vi "EnFlo_Hub.vi"() -> ()   [LabVIEW 2015]
uses:
  Anemometry Sub Vis/Controls/Launch_controls/Open_Calib.ctl
  Anemometry Sub Vis/Controls/Launch_controls/Open_Meas.ctl
  Anemometry Sub Vis/Controls/Launch_controls/Open_Enter_Temp.ctl
  Anemometry Sub Vis/Controls/Launch_controls/Multi_Run_Prog.ctl
  Anemometry Sub Vis/Controls/Launch_controls/EnFlo_arm.ctl
  Anemometry Sub Vis/Controls/Launch_controls/Fast_FID_Valve.ctl
  Anemometry Sub Vis/Controls/Launch_controls/Disp_Setup.ctl
  Anemometry Sub Vis/Controls/Launch_controls/EnFlo_Tun_Setup.ctl
  Anemometry Sub Vis/Controls/Launch_controls/User_Metadata.ctl
  Anemometry Sub Vis/Controls/Launch_controls/Trav_3D_move.ctl
  Anemometry Sub Vis/Controls/Launch_controls/Trav_Space.ctl
  Anemometry Sub Vis/Controls/Launch_controls/Tunnel_speed.ctl
  Anemometry Sub Vis/Controls/Launch_controls/Client_source_control.ctl
  Anemometry Sub Vis/Controls/Launch_controls/Hydrosonic_Manual.ctl
  Anemometry Sub Vis/Controls/Launch_controls/Preference_Panel.ctl
  Anemometry Sub Vis/Controls/Launch_controls/Hot_wire_Calculator.ctl
  Anemometry Sub Vis/Controls/Launch_controls/RW_X_Parker_Config.ctl
  Anemometry Sub Vis/Controls/Launch_controls/LDA_Alignment.ctl
  Anemometry Sub Vis/Controls/Launch_controls/Named_Serial_Comms.ctl
  Anemometry Sub Vis/Controls/Launch_controls/BSA_data_rates.ctl
  Anemometry Sub Vis/Controls/Launch_controls/Serial_Setup.ctl
  Anemometry Sub Vis/Controls/Launch_controls/Post_Process_icon.ctl
  Anemometry Sub Vis/Controls/Launch_controls/Edit_Ascii_file.ctl
  Anemometry Sub Vis/Controls/Launch_controls/Edit_Raw_DF.ctl
  Anemometry Sub Vis/Controls/Launch_controls/Results_file_plotter.ctl
  Anemometry Sub Vis/Controls/Launch_controls/Serial_Port_Names.ctl
  Anemometry Sub Vis/Controls/Launch_controls/Paul.ctl
  Anemometry Sub Vis/Controls/Launch_controls/Tom.ctl
  Anemometry Sub Vis/Controls/Launch_controls/Scani_Valve.ctl
  Anemometry Sub Vis/Controls/Launch_controls/Edit_sever_Channel.ctl
  Anemometry Sub Vis/Controls/Launch_controls/Day_file_plotter.ctl
  Anemometry Sub Vis/Controls/Launch_controls/Plot_Sever_Data.ctl
  Anemometry Sub Vis/Controls/Launch_controls/Adam_Table.ctl
  Anemometry Sub Vis/Controls/Launch_controls/Active_Channel_Control.ctl
  Anemometry Sub Vis/Controls/Launch_controls/Laser on,off.ctl
  Anemometry Sub Vis/Controls/Launch_controls/Laser set power.ctl
  Anemometry Sub Vis/Controls/Preference_Mode.ctl
  Anemometry Sub Vis/Controls/Post_Process.ctl
  Anemometry Sub Vis/Controls/Server_Comms.ctl
  ADAM Client/Sub VIs/ADAM Controls/Update_scan_value.ctl
  Anemometry Sub Vis/Controls/Setup.ctl
  Anemometry Sub Vis/Gen Trav/Trav_mode.ctl
  Anemometry Sub Vis/Controls/User_Specific_mode.ctl
  Anemometry Sub Vis/File/Setup_Filetype.ctl
  Anemometry Sub Vis/Calibration/Calib_mode.ctl
  Anemometry Sub Vis/Controls/App_Global.ctl
  Anemometry Sub Vis/Globals/Dynamic_call_global.ph.vi
  Anemometry Sub Vis/Globals/Trav_pos_global.vi
  Anemometry Sub Vis/Globals/Constants_global.vi
  Anemometry Sub Vis/Globals/Preference_global.vi
  Anemometry Sub Vis/Acquisition/PWA/PWAtasksGLOBAL.vi
  Anemometry Sub Vis/Globals/Meas_global.vi
  <vilib>/Platform/browser.llb/Open URL in Default Browser (path).vi
  <vilib>/Platform/browser.llb/Open URL in Default Browser (string).vi
  Anemometry Sub Vis/Utilities/Email_transfer_global.vi
  Camera Server/Globals/CamServer global.vi
panel:
  out "CamServer machine name or IP":string="EnFlo-CamServer"
  out "List of ADAM channels to view":string[](array[string])
  out "List of ADAM control channels":string[](array[string])
  out "Analogue Dev Name":string="Dev2"
  out "Numeric":i32
  out "Rig Name":string="EnFlo Tunnel"
  out "All Users":path=path "/System Folder/Preferences/LabVIEW (EnFlo specific)/Meas Setups"
  out "Dummy Measurement":bool
  in  "stop":bool
  in  "Tab Control":T1(tab)
  in  "Tunnel Speed Control":T2
  in  "Traverse Space":T3
  in  "Trav 3D Move":T4 caption="3D Traverse Move"
  in  "User Metadata":T5
  in  "Multi Run Prog":T6
  in  "Enter Temp_Press":T7
  in  "Measurement Prog":T8 caption="Measurement"
  in  "Calibration Prog":T9 caption="Calibration"
  in  "Source Live":bool
  in  "Laser set power":T10
  in  "Laser on/off":T11
  in  "Scani Valve":T12
  in  "LDA Alignment":T13
  in  "Hydrosonic Control":T14
  in  "Fast FID Valve":T15
  in  "Source Control":T16
  in  "Gas Release Setup":T17
  in  "EnFlo Tunnel Setup":T18
  in  "Heater Setup":bool caption="Inlet heater File"
  in  "EnFlo Arm":T19
  in  "EnFlo Tun Display":bool
  in  "Beam Check Positions":bool
  in  "Rig_Control":cluster{"Ch Name":string, "Boolean":bool}[](array[cluster])
  in  "ADAM Channels Control":T20 caption="Change Active Channels"
  in  "ADAM Scan Table":T21 caption="Run ADAM Scan Table"
  in  "Edit Server Channel":T22
  in  "Plot Server Channels":T23 caption="Plot Server Data"
  in  "Day Files Plotter":T24 caption="Plot Data From File"
  out "Current Values":cluster{"Ch Name":string, "Numeric":dbl}[](array[cluster])
  in  "Post_Pro_Results_Hierarchy":bool
  in  "Results File Plotter":T25
  in  "Edit Raw Data Files":T26
  in  "Edit ASCII File":T27
  in  "Post Process Raw Data":T28
  in  "Plot_FFID_Calibs.vi":bool
  in  "Top Level Traverse":bool
  in  "Show Manual Sync":bool
  in  "Sync to server now":bool
  in  "Port Names":T29
  in  "Serial Setup":T30
  in  "LDA Data Rate":T31
  in  "Named Serial Comms":T32
  in  "RW Trav Setup":T33
  in  "Hot Wire Calc":T34
  in  "Preference Panel":T35
  in  "Tom Lawton tlawton@cppwind.com":T36 caption="For -other- support"
  in  "Paul Hayden p.hayden@surrey.ac.uk":T37 caption="For software support"
  in  "Online Manual":bool
  out "VI Name":string
  out "Iterations":i32
  # "Or give us a call on Tel: 01483 689545"
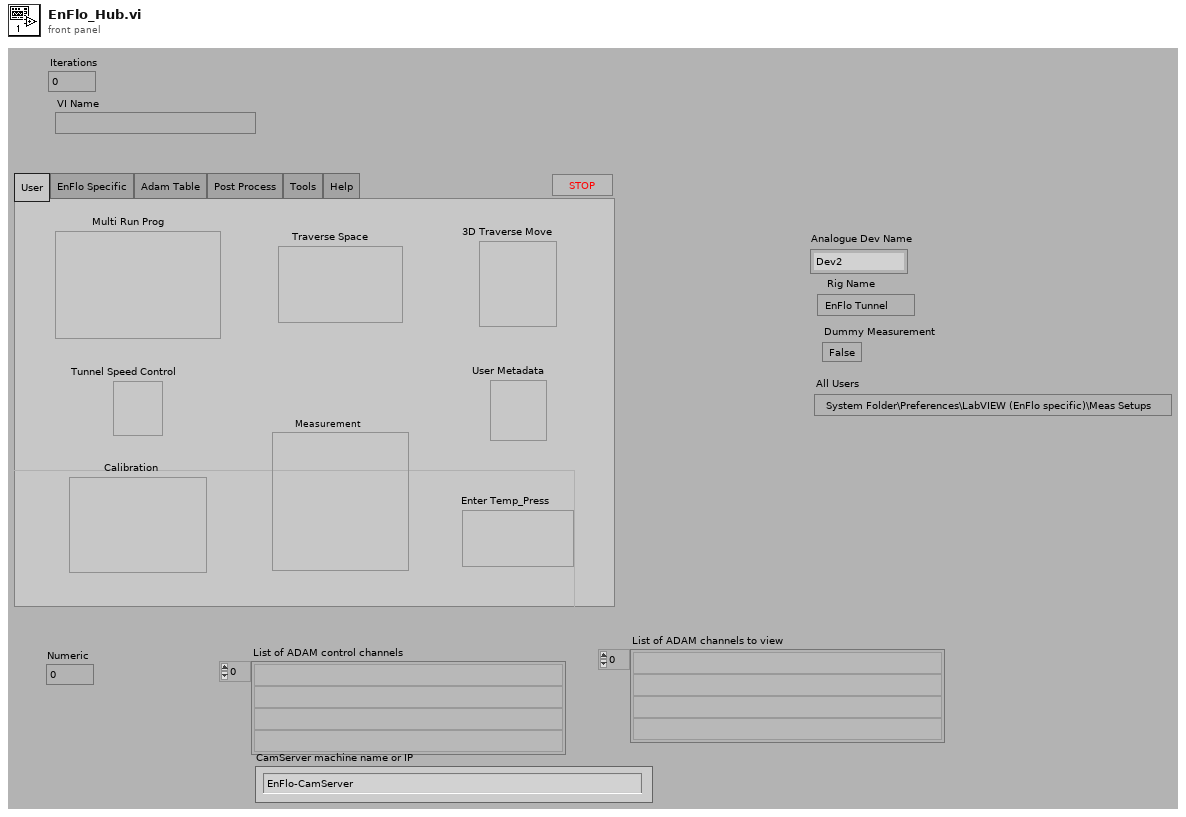
[diagram p1: front panel]
types:
  T1 = enum32{"User", "EnFlo Specific", "Adam Table", "Post Process", "Tools", "Help"}
  T2 = typedef "Tunnel_speed.ctl" = bool
  T3 = typedef "Trav_Space.ctl" = bool
  T4 = typedef "Trav_3D_move.ctl" = bool
  T5 = typedef "User_Metadata.ctl" = bool
  T6 = typedef "Multi_Run_Prog.ctl" = bool
  T7 = typedef "Open_Enter_Temp.ctl" = bool
  T8 = typedef "Open_Meas.ctl" = bool
  T9 = typedef "Open_Calib.ctl" = bool
  T10 = typedef "Laser set power.ctl" = bool
  T11 = typedef "Laser on,off.ctl" = bool
  T12 = typedef "Scani_Valve.ctl" = bool
  T13 = typedef "LDA_Alignment.ctl" = bool
  T14 = typedef "Hydrosonic_Manual.ctl" = bool
  T15 = typedef "Fast_FID_Valve.ctl" = bool
  T16 = typedef "Client_source_control.ctl" = bool
  T17 = typedef "Disp_Setup.ctl" = bool
  T18 = typedef "EnFlo_Tun_Setup.ctl" = bool
  T19 = typedef "EnFlo_arm.ctl" = bool
  T20 = typedef "Active_Channel_Control.ctl" = bool
  T21 = typedef "Adam_Table.ctl" = bool
  T22 = typedef "Edit_sever_Channel.ctl" = bool
  T23 = typedef "Plot_Sever_Data.ctl" = bool
  T24 = typedef "Day_file_plotter.ctl" = bool
  T25 = typedef "Results_file_plotter.ctl" = bool
  T26 = typedef "Edit_Raw_DF.ctl" = bool
  T27 = typedef "Edit_Ascii_file.ctl" = bool
  T28 = typedef "Post_Process_icon.ctl" = bool
  T29 = typedef "Serial_Port_Names.ctl" = bool
  T30 = typedef "Serial_Setup.ctl" = bool
  T31 = typedef "BSA_data_rates.ctl" = bool
  T32 = typedef "Named_Serial_Comms.ctl" = bool
  T33 = typedef "RW_X_Parker_Config.ctl" = bool
  T34 = typedef "Hot_wire_Calculator.ctl" = bool
  T35 = typedef "Preference_Panel.ctl" = bool
  T36 = typedef "Tom.ctl" = bool
  T37 = typedef "Paul.ctl" = bool
  T38 = typedef "Post_Process.ctl" = enum16{"Take New Data", "Post Process Raw Data File"}
  T39 = typedef "Preference_Mode.ctl" = enum16{"Load Preferences from file", "Save Preferences to file", "Load, Edit then Save"}
  T40 = enum32{"User", "EnFlo Lab Specific", "Adam Table", "Post Process", "Tools", "Help"}
  T41 = typedef "Server_Comms.ctl" = enum16{"Server Link Healthy", "Do Not Link To Server"}
  T42 = typedef "Update_scan_value.ctl" = cluster{"Channel Name":string, "New Value":dbl}
  T43 = typedef "Setup.ctl" = enum16{"Run Program", "Show Setup", "Save Current Setup", "Setup Front Panel"}
  T44 = enum16{"Get Channel Names", "Get Current Value", "Update Channel Value", "Update Channel Description"}
  T45 = enum32{"Invalid", "Standard", "Closed", "Hidden", "Minimized", "Maximized"}
  T46 = enum32{"Bad", "Idle", "Run top level", "Running"}
  T47 = enum16{"Load From Excel File", "Save to Excel File"}
  T48 = typedef "User_Specific_mode.ctl" = enum16{"Check VI only", "Run VI"}
  T49 = typedef "Trav_mode.ctl" = enum16{"Move traverse", "Read traverse position", "Teach Position"}
  T50 = typedef "Setup_Filetype.ctl" = enum16{"Measurement Setups", "Calibration Setups", "General", "Results File Plotter Setups", "Speed Calib Tweaks"}
  T51 = enum16{"Load Command File", "Save Command File", "Check Multi Run Prog", "Check Multi Run Prog With Live Moves", "Run Multi Run Prog"}
  T52 = typedef "Calib_mode.ctl" = enum16{"Show Setup", "Take a New Calibration Point", "Refit Curve", "Setup Front Panel"}
  T53 = typedef "App_Global.ctl" = enum16{"Read Global", "Write to Global", "Initialise Array"}
  T54 = typedef "Tunnel_Coordinates.ctl" = enum16{"Work in Tunnel Coordinates", "Work in Model Coordinates"}
  T55 = typedef "App_Ref_Cluster.ctl" = cluster{"Server IP & Port No":string, "Application reference":refnum<vi>}
  T56 = typedef "Ch_description_ADAM.ctl" = cluster{"Ch Name":string, "Type":T57, "Function":T58, "Ch State":T59, "Calibration type":T60, "A":dbl, "B":dbl, "C":dbl, "D":dbl, "Comments":string, "Address":T61, "String":string, "Duty":u16}
  T57 = typedef "Module_type_ADAM.ctl" = string
  T58 = typedef "Function_ADAM.ctl" = enum16{"Analogue Input", "Digital Input", "Event counter", "Event rate", "Analogue Output", "Digital Output", "Relay Output"}
  T59 = typedef "Channel_State.ctl" = enum16{"On", "Off", "Always On", "Always Off"}
  T60 = typedef "Calib_type_ADAM.ctl" = enum16{"Raw", "Bx + A", "Cx^2 + Bx + A", "Dx^3 + Cx^2 + Bx + A", "In Band", "Hi-Tec Q", "Hi-Tec M_dot", "Text"}
  T61 = typedef "Address.ctl" = cluster{"Main":i32, "Ch.":i32, "Sub":i32, "Port Name":string}
  T62 = typedef "Monitor values.ctl" = cluster{"Power (mW)":sgl, "LDD current (A)":sgl, "TEC drive (V)":sgl, "TEC temp. (degC)":sgl, "SHG heater (degC)":sgl, "BRF heater (degC)":sgl}
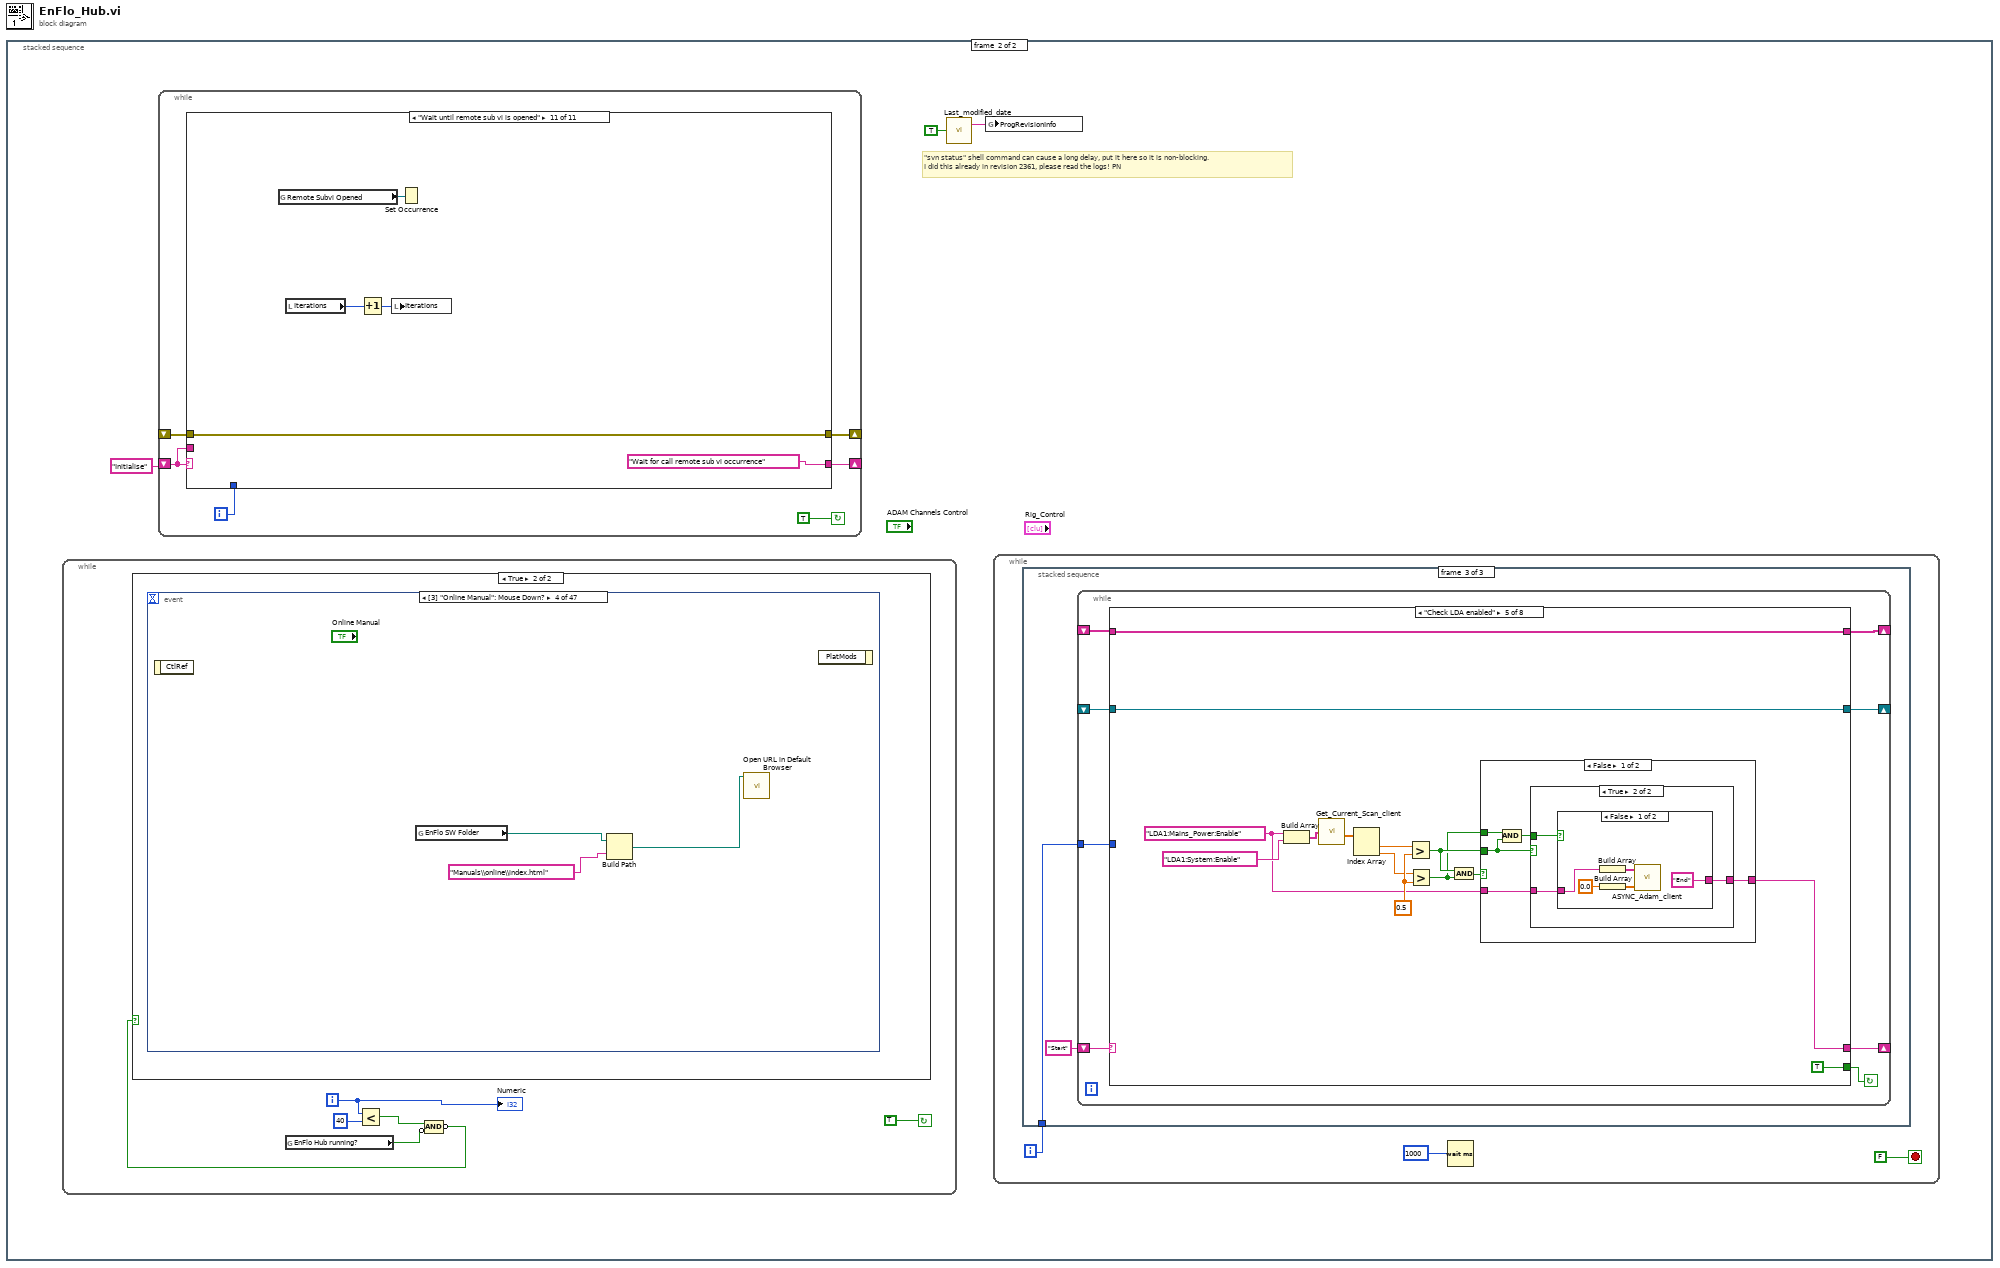
[diagram p0: block diagram]
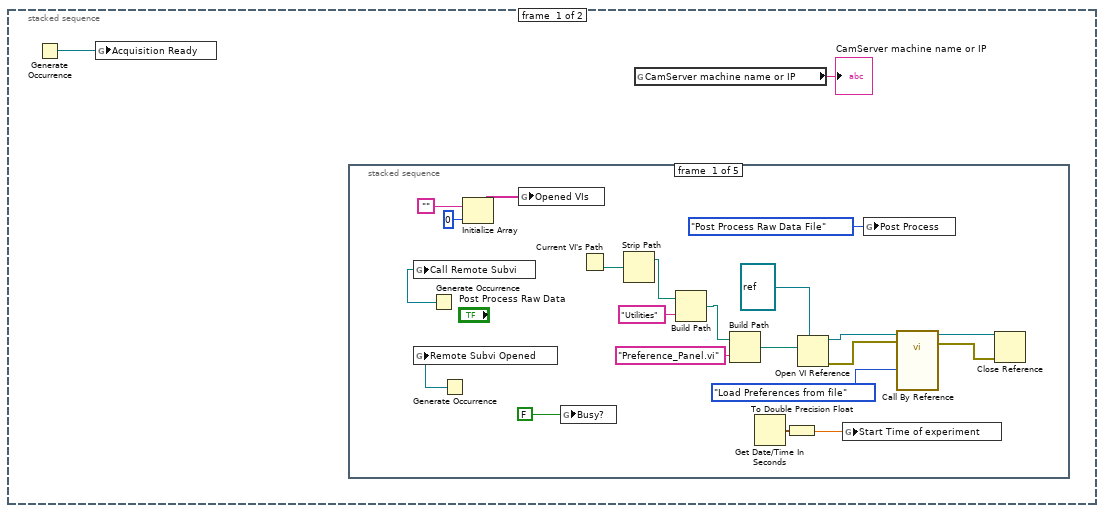
[diagram p2: hidden frame]
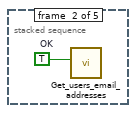
[diagram p3: hidden frame]
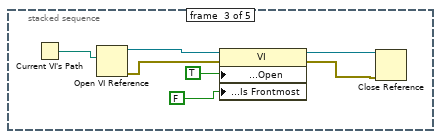
[diagram p4: hidden frame]
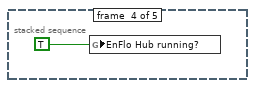
[diagram p5: hidden frame]
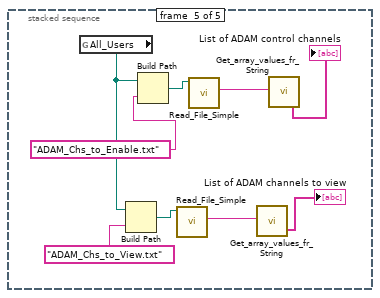
[diagram p6: hidden frame]
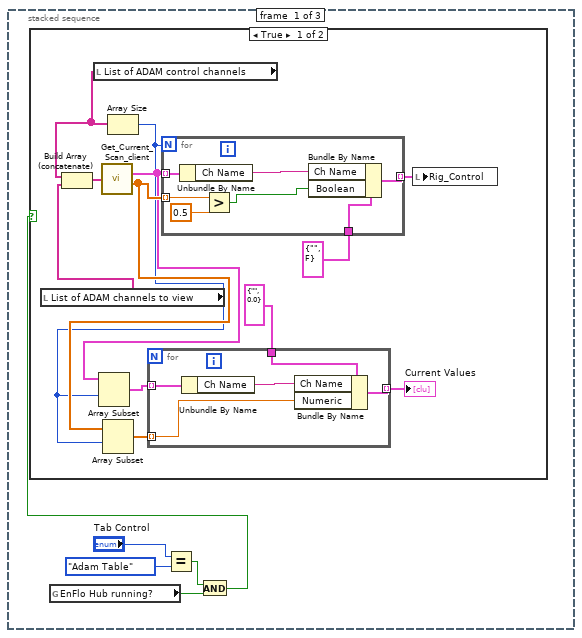
[diagram p7: hidden frame]
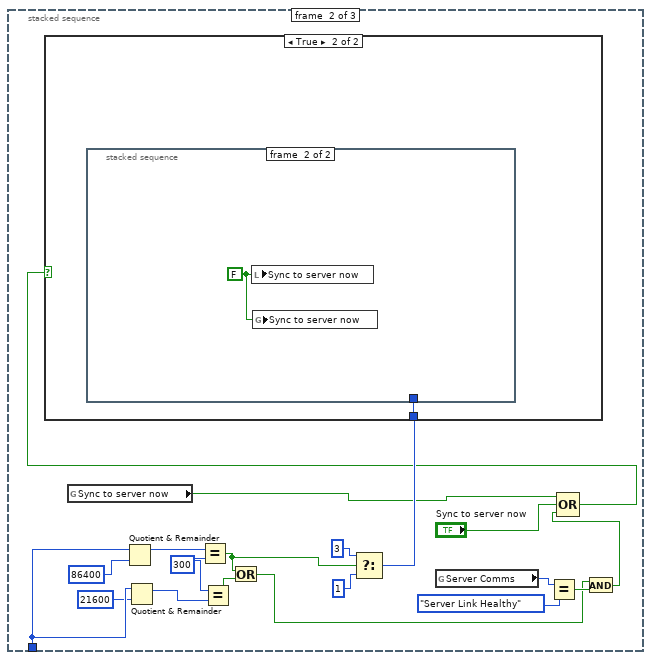
[diagram p9: hidden frame]
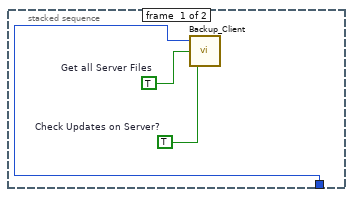
[diagram p11: hidden frame]
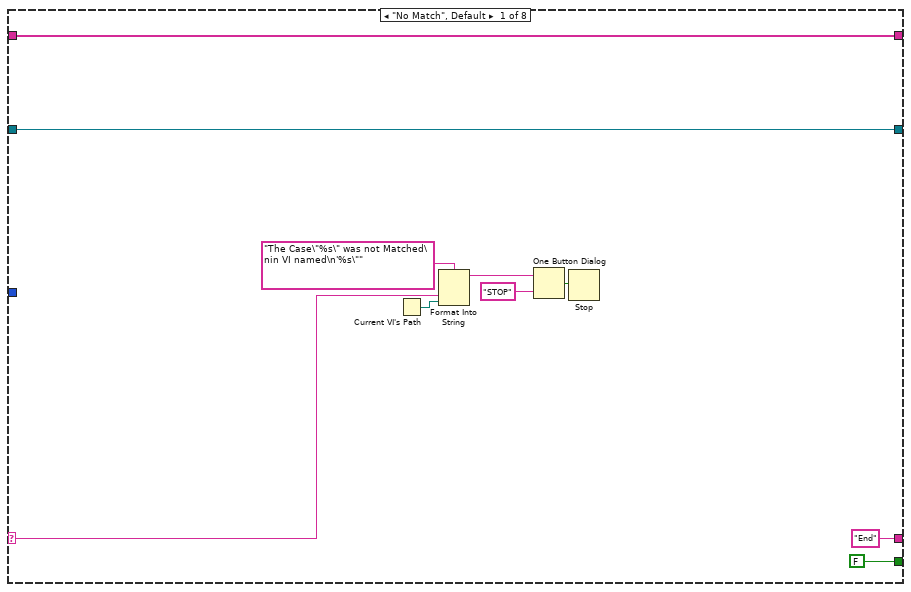
[diagram p12: hidden frame]
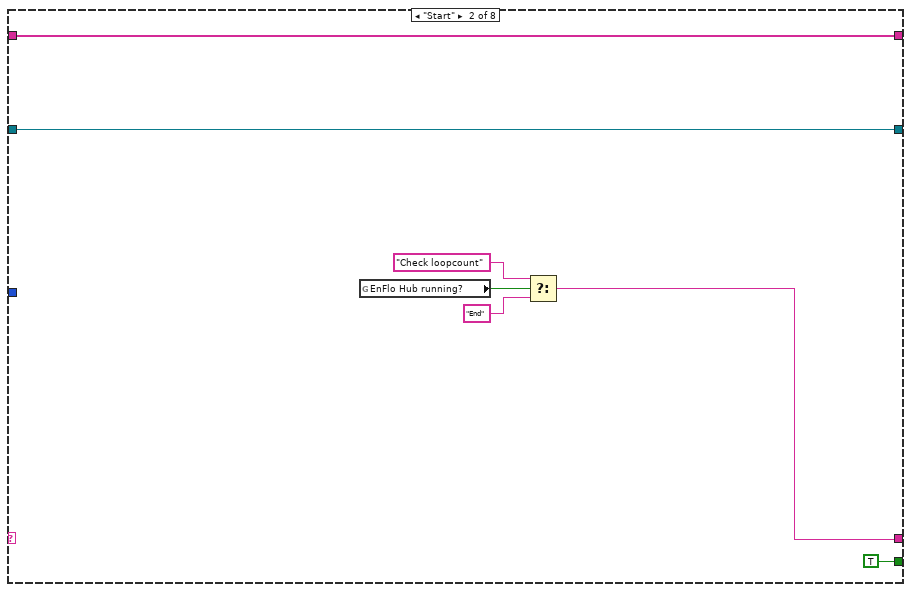
[diagram p13: hidden frame]
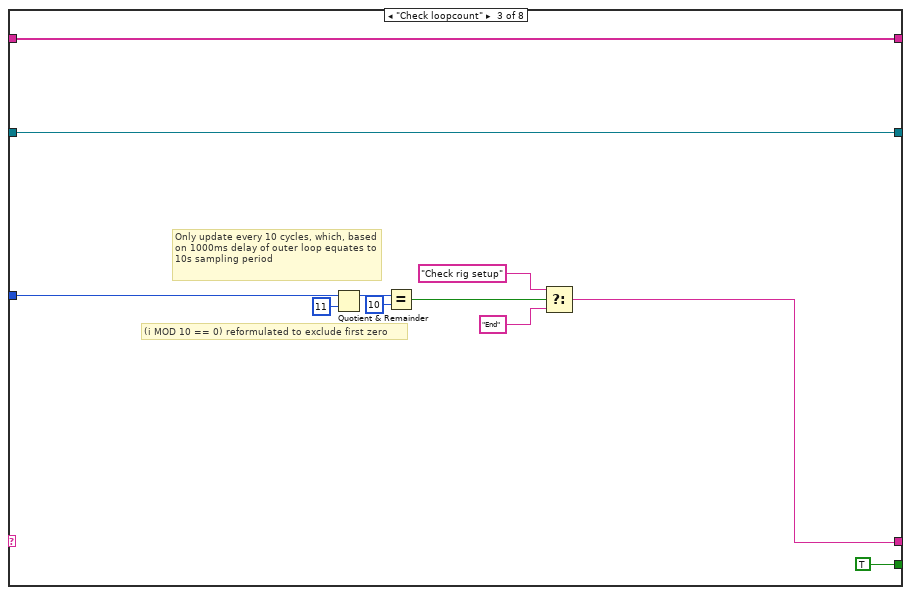
[diagram p14: hidden frame]
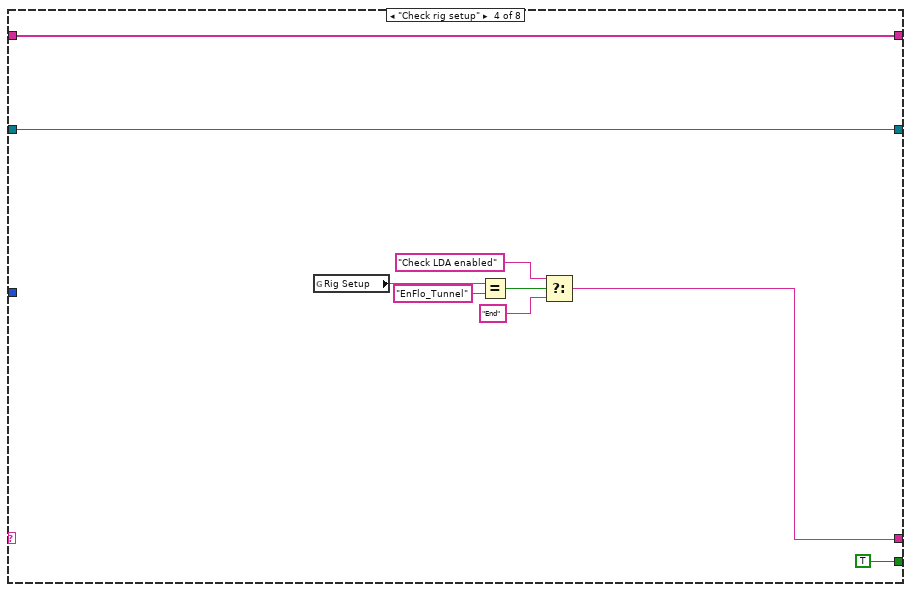
[diagram p15: hidden frame]
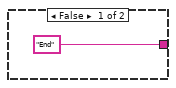
[diagram p16: hidden frame]
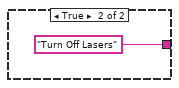
[diagram p17: hidden frame]
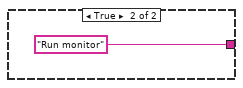
[diagram p18: hidden frame]
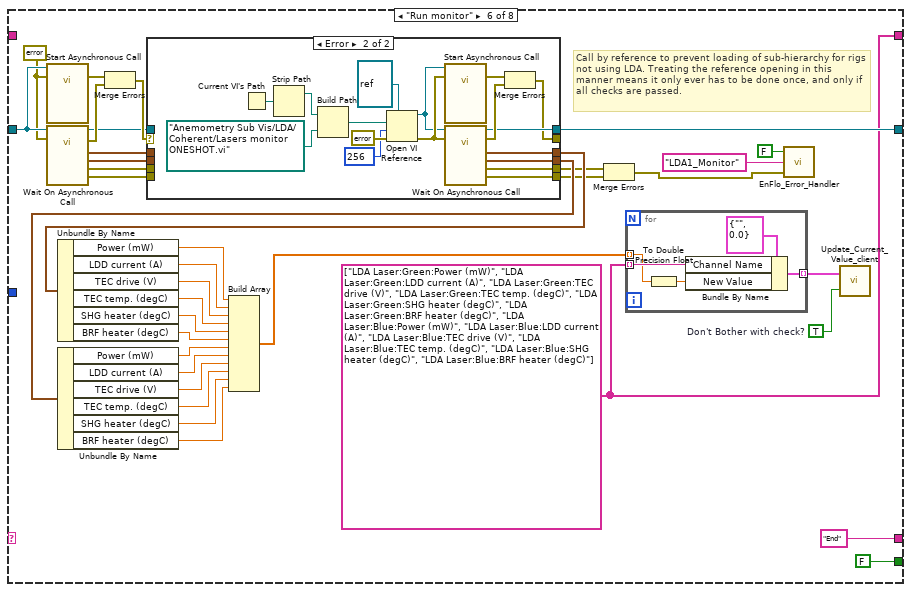
[diagram p19: hidden frame]
diagram:
  n1 = stacked-sequence {
    frame #0 {
      n2 = Generate Occurrence() -> (w2:refnum<k4>)
      n3 = global write "Meas_global.vi" "Acquisition Ready"(w2) -> ()
      n4 = stacked-sequence {
        frame #0 {
          n5 = Generate Occurrence() -> (w23:refnum<k4>)
          n6 = global write "Dynamic_call_global.ph.vi" "Call Remote Subvi"(w23) -> ()
          n7 = Generate Occurrence() -> (w22:refnum<k4>)
          n8 = global write "Dynamic_call_global.ph.vi" "Remote Subvi Opened"(w22) -> ()
          n9 = Initialize Array("", 0) -> (w20:string[])
          n10 = global write "Dynamic_call_global.ph.vi" "Opened VIs"(w20) -> ()
          n11 = global write "Email_transfer_global.vi" "Busy?"(FALSE ("Busy?")) -> ()
          n12 = Current VI's Path() -> (path=w12:path)
          n13 = Strip Path(path=w12) -> (stripped path=w10:path)  [unwired: 1 out]
          n14 = Build Path(base path=w10, name or relative path="Utilities") -> (appended path=w8:path)
          n15 = Build Path(base path=w8, name or relative path="Preference_Panel.vi") -> (appended path=w7:path)
          n16 = Get Date/Time In Seconds() -> (seconds since 1Jan1904=w18:timestamp)
          n17 = To Double Precision Float(number=w18) -> (double precision float=w17:dbl)
          n18 = Open VI Reference(type specifier VI Refnum (for type only)=refnum<vi> refnum, vi path=w7) -> (vi reference=w13:refnum<vi>, error out=w14:errorcluster)  [unwired: 1 in, 3 out]
          n19 = global write "Meas_global.vi" "Start Time of experiment"(w17) -> ()
          n20 = global write "Meas_global.vi" "Post Process"(Post_Process."Post Process Raw Data File" ("Post Process")) -> ()
          n21 = call-by-ref "?"(reference=w13, error in=w14, "Mode"=Preference_Mode."Load Preferences from file") -> (reference out=w15:refnum<vi>, error out=w16:errorcluster)
          n22 = Close Reference(reference=w15, error in (no error)=w16) -> ()  [unwired: 1 out]
        }
        frame #1 {
          w24 = TRUE  # OK
          n23 = call "Get_users_email_addresses.vi"("OK"=w24) -> ()  [unwired: 5 out]
        }
        frame #2 {
          n24 = Current VI's Path() -> (path=w31:path)
          n25 = Open VI Reference(vi path=w31) -> (vi reference=w30:refnum<vi>, error out=w29:errorcluster)  [unwired: 1 in, 4 out]
          n26 = property class="VI"(reference=w30, error in=w29, "Front Panel Window:Open"=TRUE, "Front Panel Window:Is Frontmost"=FALSE) -> (reference out=w28:refnum<vi>, error out=w27:errorcluster)
          n27 = Close Reference(reference=w28, error in (no error)=w27) -> ()  [unwired: 1 out]
        }
        frame #3 {
          n28 = global write "Dynamic_call_global.ph.vi" "EnFlo Hub running?"(TRUE ("EnFlo Hub running?")) -> ()
        }
        frame #4 {
          n29 = global read "Constants_global.vi" "All_Users"() -> (w36:path)
          n30 = Build Path(base path=w36, name or relative path="ADAM_Chs_to_View.txt") -> (appended path=w38:path)
          n31 = Build Path(base path=w36, name or relative path="ADAM_Chs_to_Enable.txt") -> (appended path=w40:path)
          n32 = call "Read_File_Simple.vi"("Filename"=w38) -> ("string"=w37:string)  [unwired: 2 in, 7 out]
          n33 = call "Read_File_Simple.vi"("Filename"=w40) -> ("string"=w41:string)  [unwired: 2 in, 7 out]
          n34 = call "Get_array_values_fr_String.vi"("String Value"=w37) -> ("String array"=→"List of ADAM channels to view":string[])  [unwired: 1 out]
          n35 = call "Get_array_values_fr_String.vi"("String Value"=w41) -> ("String array"=→"List of ADAM control channels":string[])  [unwired: 1 out]
        }
      }
      n36 = global read "CamServer global.vi" "CamServer machine name or IP"() -> (→"CamServer machine name or IP":string)
    }
    frame #1 {
      # "\"svn status\" shell command can cause a long delay, put it here so it is non-blocking.\nI did this already in revision 2361, please read the logs! PN"
      n37 = while {
        i -> [w272]
        stop <- TRUE continue-if-true
        n38 = global read "Dynamic_call_global.ph.vi" "EnFlo Hub running?"() -> (w270:bool)
        n39 = Less?(x=w272, y=40) -> (x < y?=w269:bool)
        n40 = Compound Arithmetic op=AND(w269, invert w270) -> (invert w268:bool)
        n41 = case shown="True" w268 {
          frame False {
            n42 = Wait (ms)(milliseconds to wait=u32 200) -> ()  [unwired: 1 out]
          }
          frame True {
            n43 = event shown="[3] \"Online Manual\": Mouse Down?" {
              selector: _ -> [_ _ _ _ _ _ _ _ _ _ _ _ _ _ _ _ _ _ _ _ _ _ _ _ _ _ _ _ _ _ _ _ _ _ _ _ _ _ _ _ _ _ _ _ _ _ _]
              dyn-events: _ -> [_ _ _ _ _ _ _ _ _ _ _ _ _ _ _ _ _ _ _ _ _ _ _ _ _ _ _ _ _ _ _ _ _ _ _ _ _ _ _ _ _ _ _ _ _ _ _]
              timeout: _ -> [_ _ _ _ _ _ _ _ _ _ _ _ _ _ _ _ _ _ _ _ _ _ _ _ _ _ _ _ _ _ _ _ _ _ _ _ _ _ _ _ _ _ _ _ _ _ _]
              event Mouse Down? {
                w283 = "Measurement.vi" ("name or relative path")
                n44 = event-data() -> ()  [unwired: 2 out]
                n45 = global read "Constants_global.vi" "EnFlo SW Folder"() -> (w286:path)
                n46 = Open VI Reference(vi path=w283) -> (vi reference=w282:refnum<vi>, error out=w281:errorcluster)  [unwired: 1 in, 4 out]
                n47 = Build Path(base path=w286, name or relative path="Anemometry") -> (appended path=w289:path)
                n48 = property class="VI"(reference=w282, error in=w281, "Front Panel Window:Open"=TRUE) -> (reference out=w279:refnum<vi>, error out=w280:errorcluster)
                n49 = Build Path(base path=w289, name or relative path=w283) -> (appended path=w287:path)
                n50 = global read "Preference_global.vi" "Rig Setup"() -> (w277:string)
                n51 = Close Reference(reference=w279, error in (no error)=w280) -> (error out=w278:errorcluster)
                n52 = Unbundle By Name(w278) -> ("status"=w288:bool)
                n53 = Equal?(x="Post_Processing_Machine" ("Rig Setup"), y=w277) -> (x = y?=w275:bool)
                n54 = case shown="True" w288 {
                  tunnel: w287 -> [_ w292]
                  tunnel: w278 -> [_ _]
                  tunnel: w275 -> [_ w291]
                  frame False {
                  }
                  frame True {
                    n55 = stacked-sequence {
                      tunnel: w292 -> [w302 _]
                      tunnel: w291 -> [w293 _]
                      frame #0 {
                        n56 = Open VI Reference(type specifier VI Refnum (for type only)=refnum<vi> refnum, vi path=w302) -> (vi reference=w300:refnum<vi>, error out=w299:errorcluster)  [unwired: 1 in, 3 out]
                        n57 = property class="VI Interface Type 2"(reference=w300, error in=w299, "Front Panel Window:Open"=TRUE) -> (reference out=w295:refnum<vi>, error out=w294:errorcluster)
                        n58 = case shown="False" w293 {
                          tunnel: [w308 w310] -> w298
                          tunnel: [w307 w309] -> w297
                          tunnel: w295 -> [w306 w310]
                          tunnel: w294 -> [w305 w309]
                          frame False {
                            n59 = call-by-ref "?"(reference=w306, error in=w305, "setup"=Setup."Setup Front Panel", "Post Process"=Post_Process."Take New Data") -> (reference out=w308:refnum<vi>, error out=w307:errorcluster)  [unwired: 16 in, 2 out]
                          }
                          frame True {
                          }
                        }
                        n60 = Close Reference(reference=w298, error in (no error)=w297) -> ()  [unwired: 1 out]
                      }
                      frame #1 {
                        n61 = global write "Meas_global.vi" "Post Process"(Post_Process."Post Process Raw Data File" ("Post Process")) -> ()
                      }
                    }
                  }
                }
                n62 = event-data("Discard?"=TRUE) -> ()  [unwired: 1 in, 2 out]
              }
              event Mouse Down? {
                n63 = event-data() -> ()  [unwired: 2 out]
                n64 = call-poly <vilib>:"Open URL in Default Browser.vi"("URL"="Mailto:tlawton@cppwind.com") -> ()  [unwired: 1 in, 6 out]
                n65 = event-data() -> ()  [unwired: 1 in, 5 out]
              }
              event Mouse Down? {
                n66 = event-data() -> ()  [unwired: 5 out]
                n67 = call-poly <vilib>:"Open URL in Default Browser.vi"("URL"="Mailto:p.hayden@surrey.ac.uk") -> ()  [unwired: 1 in, 6 out]
                n68 = event-data() -> ()  [unwired: 1 in, 2 out]
              }
              event "Online Manual": Mouse Down? {
                n69 = event-data() -> ()  [unwired: 2 out]
                n70 = global read "Constants_global.vi" "EnFlo SW Folder"() -> (w316:path)
                n71 = Build Path(base path=w316, name or relative path="Manuals\\online\\index.html" ("URL")) -> (appended path=w314:path)
                n72 = call-poly <vilib>:"Open URL in Default Browser.vi"("path"=w314) -> ()  [unwired: 1 in, 6 out]
                n73 = event-data() -> ()  [unwired: 1 in, 2 out]
              }
              event Mouse Down? {
                n74 = event-data() -> ()  [unwired: 9 out]
                n75 = global read "Constants_global.vi" "EnFlo SW Folder"() -> (w317:path)
                n76 = Build Path(base path=w317, name or relative path=path "ADAM Client/ADAM client VIs/ScaniValve_client.vi") -> (appended path=w320:path)
                n77 = call "Open_Close_Front_Panel.ph.vi"("Front Panel Window:Open"=TRUE, "VI path"=w320) -> ()  [unwired: 2 out]
                n78 = event-data() -> ()  [unwired: 1 in, 5 out]
              }
              event Mouse Down? {
                n79 = event-data() -> ()  [unwired: 9 out]
                n80 = global read "Constants_global.vi" "EnFlo SW Folder"() -> (w321:path)
                n81 = Build Path(base path=w321, name or relative path=path "Anemometry/Anemometry Sub Vis/LDA/Coherent/Laser power on,off (simple).vi") -> (appended path=w324:path)
                n82 = call "Open_Close_Front_Panel.ph.vi"("Front Panel Window:Open"=TRUE, "VI path"=w324) -> ()  [unwired: 2 out]
                n83 = event-data() -> ()  [unwired: 2 in, 1 out]
              }
              event "Source Live": Value Change {
                n84 = event-data() -> ()  [unwired: 7 out]
                n85 = flat-sequence {
                  frame #0 {
                    n86 = global read "Constants_global.vi" "EnFlo SW Folder"() -> (w325:path)
                    n87 = Build Path(base path=w325, name or relative path=path "ADAM Serial/Instrument drivers/Arduino/Source_Live_Control.vi") -> (appended path=w328:path)
                    n88 = call "Open_Close_Front_Panel.ph.vi"("Front Panel Window:Open"=TRUE, "VI path"=w328) -> ()  [unwired: 2 out]
                  }
                  frame #1 {
                    n89 = local write "Source Live"(FALSE) -> ()
                  }
                }
              }
              event Mouse Down? {
                n90 = event-data() -> ()  [unwired: 9 out]
                n91 = global read "Constants_global.vi" "EnFlo SW Folder"() -> (w330:path)
                n92 = Build Path(base path=w330, name or relative path=path "Anemometry/Anemometry Sub Vis/LDA/Coherent/Set lasers power.vi") -> (appended path=w333:path)
                n93 = call "Open_Close_Front_Panel.ph.vi"("Front Panel Window:Open"=TRUE, "VI path"=w333) -> ()  [unwired: 2 out]
                n94 = event-data() -> ()  [unwired: 2 in, 1 out]
              }
              event Mouse Down? {
                n95 = event-data() -> ()  [unwired: 5 out]
                n96 = global read "Constants_global.vi" "EnFlo SW Folder"() -> (w334:path)
                n97 = Build Path(base path=w334, name or relative path=path "ADAM Client/ADAM client VIs/Day_File_Plotter.vi") -> (appended path=w340:path)
                n98 = Open VI Reference(vi path=w340) -> (vi reference=w341:refnum<vi>, error out=w343:errorcluster)  [unwired: 2 in, 3 out]
                n99 = property class="VI"(reference=w341, error in=w343, "Front Panel Window:Open"=TRUE) -> (reference out=w345:refnum<vi>, error out=w344:errorcluster)
                n100 = invoke class="VI" method="Run VI"(reference=w345, error in=w344, "Wait until done"=FALSE, "Auto Dispose Ref"=TRUE) -> (reference out=w336:refnum<vi>, error out=w337:errorcluster)  [unwired: 1 in, 3 out]
                n101 = Close Reference(reference=w336, error in (no error)=w337) -> ()  [unwired: 1 out]
                n102 = event-data() -> ()  [unwired: 1 in, 4 out]
              }
              event Mouse Down? {
                n103 = event-data() -> ()  [unwired: 5 out]
                n104 = global read "Constants_global.vi" "EnFlo SW Folder"() -> (w346:path)
                n105 = Build Path(base path=w346, name or relative path=path "ADAM Serial/Serial Link Layer/Port_Names.vi") -> (appended path=w348:path)
                n106 = Open VI Reference(vi path=w348) -> (vi reference=w353:refnum<vi>, error out=w354:errorcluster)  [unwired: 1 in, 4 out]
                n107 = invoke class="VI" method="Run VI"(reference=w353, error in=w354, "Wait until done"=TRUE, "Auto Dispose Ref"=TRUE) -> (reference out=w349:refnum<vi>, error out=w350:errorcluster)  [unwired: 1 in, 3 out]
                n108 = Close Reference(reference=w349, error in (no error)=w350) -> ()  [unwired: 1 out]
                n109 = event-data() -> ()  [unwired: 1 in, 5 out]
              }
              event Mouse Down? {
                n110 = event-data() -> ()  [unwired: 5 out]
                n111 = global read "Constants_global.vi" "EnFlo SW Folder"() -> (w355:path)
                n112 = Build Path(base path=w355, name or relative path=path "Data plotting/Results_file_Plotter.vi") -> (appended path=w358:path)
                n113 = Open VI Reference(vi path=w358) -> (vi reference=w360:refnum<vi>, error out=w357:errorcluster)  [unwired: 1 in, 4 out]
                n114 = property class="VI"(reference=w360, error in=w357, "Front Panel Window:Open"=TRUE) -> (reference out=w361:refnum<vi>, error out=w362:errorcluster)
                n115 = invoke class="VI" method="Run VI"(reference=w361, error in=w362, "Wait until done"=FALSE, "Auto Dispose Ref"=TRUE) -> (reference out=w363:refnum<vi>, error out=w364:errorcluster)  [unwired: 1 in, 3 out]
                n116 = Close Reference(reference=w363, error in (no error)=w364) -> ()  [unwired: 1 out]
                n117 = event-data() -> ()  [unwired: 1 in, 5 out]
              }
              event Mouse Down? {
                n118 = event-data() -> ()  [unwired: 5 out]
                n119 = global read "Constants_global.vi" "EnFlo SW Folder"() -> (w367:path)
                n120 = Build Path(base path=w367, name or relative path=path "Anemometry/Utilities/Post_Process_Raw_data.vi") -> (appended path=w369:path)
                n121 = call "Open_Close_Front_Panel.ph.vi"("Front Panel Window:Open"=TRUE, "VI path"=w369) -> ()  [unwired: 2 out]
                n122 = event-data() -> ()  [unwired: 1 in, 5 out]
              }
              event Mouse Down? {
                n123 = event-data() -> ()  [unwired: 5 out]
                n124 = global read "Constants_global.vi" "EnFlo SW Folder"() -> (w371:path)
                n125 = Build Path(base path=w371, name or relative path=path "Anemometry/Anemometry Sub Vis/Data_plotting_vis/Edit_Raw_DF_Header.vi") -> (appended path=w373:path)
                n126 = call "Open_Close_Front_Panel.ph.vi"("Front Panel Window:Open"=TRUE, "VI path"=w373) -> ()  [unwired: 2 out]
                n127 = event-data() -> ()  [unwired: 1 in, 5 out]
              }
              event Mouse Down? {
                n128 = event-data() -> ()  [unwired: 5 out]
                n129 = global read "Constants_global.vi" "EnFlo SW Folder"() -> (w375:path)
                n130 = Build Path(base path=w375, name or relative path=path "ADAM Serial/Serial Link Layer/Serial_Setup.vi") -> (appended path=w377:path)
                n131 = Open VI Reference(vi path=w377) -> (vi reference=w382:refnum<vi>, error out=w383:errorcluster)  [unwired: 1 in, 4 out]
                n132 = invoke class="VI" method="Run VI"(reference=w382, error in=w383, "Wait until done"=TRUE, "Auto Dispose Ref"=TRUE) -> (reference out=w378:refnum<vi>, error out=w379:errorcluster)  [unwired: 1 in, 3 out]
                n133 = Close Reference(reference=w378, error in (no error)=w379) -> ()  [unwired: 1 out]
                n134 = event-data() -> ()  [unwired: 1 in, 2 out]
              }
              event Mouse Down? {
                n135 = event-data() -> ()  [unwired: 5 out]
                n136 = global read "Constants_global.vi" "EnFlo SW Folder"() -> (w385:path)
                n137 = Build Path(base path=w385, name or relative path=path "ADAM Serial/Serial Link Layer/Named_Serial_Comms.vi") -> (appended path=w387:path)
                n138 = call "Open_Close_Front_Panel.ph.vi"("Front Panel Window:Open"=TRUE, "VI path"=w387) -> ()  [unwired: 2 out]
                n139 = event-data() -> ()  [unwired: 1 in, 5 out]
              }
              event Mouse Down? {
                n140 = event-data() -> ()  [unwired: 5 out]
                n141 = global read "Constants_global.vi" "EnFlo SW Folder"() -> (w388:path)
                n142 = Build Path(base path=w388, name or relative path=path "Anemometry/Anemometry Sub Vis/LDA/LDA_data_rate.vi") -> (appended path=w390:path)
                n143 = call "Open_Close_Front_Panel.ph.vi"("Front Panel Window:Open"=TRUE, "VI path"=w390) -> ()  [unwired: 2 out]
                n144 = event-data() -> ()  [unwired: 1 in, 2 out]
              }
              event Mouse Down? {
                n145 = event-data() -> ()  [unwired: 5 out]
                n146 = global read "Constants_global.vi" "EnFlo SW Folder"() -> (w402:path)
                n147 = Build Path(base path=w402, name or relative path=path "ADAM Client/ADAM client VIs/Control_Channel_Status.vi") -> (appended path=w392:path)
                n148 = Open VI Reference(vi path=w392) -> (vi reference=w395:refnum<vi>, error out=w393:errorcluster)  [unwired: 1 in, 4 out]
                n149 = property class="VI"(reference=w395, error in=w393, "Front Panel Window:Open"=TRUE) -> (reference out=w396:refnum<vi>, error out=w397:errorcluster)
                n150 = invoke class="VI" method="Run VI"(reference=w396, error in=w397, "Wait until done"=FALSE, "Auto Dispose Ref"=TRUE) -> (reference out=w398:refnum<vi>, error out=w399:errorcluster)  [unwired: 1 in, 3 out]
                n151 = Close Reference(reference=w398, error in (no error)=w399) -> ()  [unwired: 1 out]
                n152 = event-data() -> ()  [unwired: 1 in, 2 out]
              }
              event Mouse Down? {
                n153 = event-data() -> ()  [unwired: 5 out]
                n154 = global read "Constants_global.vi" "EnFlo SW Folder"() -> (w404:path)
                n155 = Build Path(base path=w404, name or relative path=path "Anemometry/Utilities/LDA_Beam_Alignment.vi") -> (appended path=w406:path)
                n156 = call "Open_Close_Front_Panel.ph.vi"("Front Panel Window:Open"=TRUE, "VI path"=w406) -> ()  [unwired: 2 out]
                n157 = event-data() -> ()  [unwired: 1 in, 5 out]
              }
              event Mouse Down? {
                w409 = FALSE  # Wait until done
                n158 = event-data() -> ()  [unwired: 5 out]
                n159 = call "Run_Enter_Temp.vi"("Wait until done"=w409) -> ()  [unwired: 1 out]
                n160 = event-data("Discard?"=TRUE) -> ()  [unwired: 1 in, 4 out]
              }
              event Mouse Down? {
                n161 = event-data() -> ()  [unwired: 5 out]
                n162 = global read "Constants_global.vi" "EnFlo SW Folder"() -> (w410:path)
                n163 = Build Path(base path=w410, name or relative path=path "Anemometry/Utilities/Edit_ASCI_file.vi") -> (appended path=w413:path)
                n164 = call "Open_Close_Front_Panel.ph.vi"("Front Panel Window:Open"=TRUE, "VI path"=w413) -> ()  [unwired: 2 out]
                n165 = event-data() -> ()  [unwired: 1 in, 5 out]
              }
              event "Heater Setup": Mouse Down? {
                n166 = event-data() -> ()  [unwired: 5 out]
                n167 = global read "Constants_global.vi" "EnFlo SW Folder"() -> (w414:path)
                n168 = Build Path(base path=w414, name or relative path=path "Anemometry/Utilities/Create_Heater_Setpoints_File.vi") -> (appended path=w417:path)
                n169 = call "Open_Close_Front_Panel.ph.vi"("Front Panel Window:Open"=TRUE, "VI path"=w417) -> ()  [unwired: 2 out]
                n170 = event-data() -> ()  [unwired: 1 in, 5 out]
              }
              event Mouse Down? {
                n171 = event-data() -> ()  [unwired: 5 out]
                n172 = global read "Constants_global.vi" "EnFlo SW Folder"() -> (w418:path)
                n173 = Build Path(base path=w418, name or relative path=path "ADAM Client/Sub VIs/Gas_Release_Control.vi") -> (appended path=w421:path)
                n174 = call "Open_Close_Front_Panel.ph.vi"("Front Panel Window:Open"=TRUE, "VI path"=w421) -> ()  [unwired: 2 out]
                n175 = event-data() -> ()  [unwired: 1 in, 5 out]
              }
              event Mouse Down? {
                n176 = event-data() -> ()  [unwired: 5 out]
                n177 = global read "Constants_global.vi" "EnFlo SW Folder"() -> (w422:path)
                n178 = Build Path(base path=w422, name or relative path=path "ADAM Client/ADAM client VIs/Edit_Server_Channel.vi") -> (appended path=w432:path)
                n179 = Open VI Reference(type specifier VI Refnum (for type only)=refnum<vi> refnum, vi path=w432) -> (vi reference=w425:refnum<vi>, error out=w426:errorcluster)  [unwired: 1 in, 3 out]
                n180 = property class="VI Interface Type 3"(reference=w425, error in=w426, "Front Panel Window:Open"=TRUE) -> (reference out=w428:refnum<vi>, error out=w429:errorcluster)
                n181 = call-by-ref "?"(reference=w428, error in=w429, "Mode"=T44."Get Channel Names") -> (reference out=w430:refnum<vi>, error out=w431:errorcluster)  [unwired: 5 in]
                n182 = Close Reference(reference=w430, error in (no error)=w431) -> ()  [unwired: 1 out]
                n183 = event-data() -> ()  [unwired: 1 in, 5 out]
              }
              event "EnFlo Tun Display": Mouse Down? {
                n184 = event-data() -> ()  [unwired: 9 out]
                n185 = global read "Constants_global.vi" "EnFlo SW Folder"() -> (w445:path)
                n186 = Build Path(base path=w445, name or relative path=path "Anemometry/Utilities/EnFlo_Tunnel_Display.vi") -> (appended path=w440:path)
                n187 = Open VI Reference(vi path=w440) -> (vi reference=w439:refnum<vi>, error out=w438:errorcluster)  [unwired: 5 in]
                n188 = invoke class="VI" method="FP.Open"(reference=w439, error in=w438, "Activate"=TRUE ("Activate?"), "State"=T45."Standard") -> (reference out=w437:refnum<vi>, error out=w436:errorcluster)  [unwired: 1 in, 3 out]
                n189 = invoke class="VI" method="Run VI"(reference=w437, error in=w436, "Wait until done"=FALSE ("Wait Until Done"), "Auto Dispose Ref"=FALSE ("Wait until done")) -> (reference out=w441:refnum<vi>, error out=w442:errorcluster)  [unwired: 1 in, 3 out]
                n190 = Close Reference(reference=w441, error in (no error)=w442) -> ()  [unwired: 1 out]
                n191 = event-data() -> ()  [unwired: 5 in, 1 out]
              }
              event Mouse Down? {
                n192 = event-data() -> ()  [unwired: 5 out]
                n193 = global read "Constants_global.vi" "EnFlo SW Folder"() -> (w447:path)
                n194 = Build Path(base path=w447, name or relative path=path "ADAM Client/ADAM client VIs/Set_Tunnel_Speed.vi") -> (appended path=w450:path)
                n195 = call "Open_Close_Front_Panel.ph.vi"("Front Panel Window:Open"=TRUE, "VI path"=w450) -> ()  [unwired: 2 out]
                n196 = event-data() -> ()  [unwired: 1 in, 5 out]
              }
              event Mouse Down? {
                n197 = event-data() -> ()  [unwired: 5 out]
                n198 = global read "Constants_global.vi" "EnFlo SW Folder"() -> (w451:path)
                n199 = Build Path(base path=w451, name or relative path=path "ADAM Client/ADAM client VIs/Plot_Server_Data.vi") -> (appended path=w454:path)
                n200 = Open VI Reference(vi path=w454) -> (vi reference=w456:refnum<vi>, error out=w453:errorcluster)  [unwired: 1 in, 4 out]
                n201 = property class="VI"(reference=w456, error in=w453, "Front Panel Window:Open"=TRUE) -> (reference out=w457:refnum<vi>, error out=w458:errorcluster)
                n202 = invoke class="VI" method="Run VI"(reference=w457, error in=w458, "Wait until done"=FALSE, "Auto Dispose Ref"=TRUE) -> (reference out=w459:refnum<vi>, error out=w460:errorcluster)  [unwired: 1 in, 3 out]
                n203 = Close Reference(reference=w459, error in (no error)=w460) -> ()  [unwired: 1 out]
                n204 = event-data() -> ()  [unwired: 1 in, 5 out]
              }
              event Mouse Down? {
                n205 = event-data() -> ()  [unwired: 5 out]
                n206 = global read "Constants_global.vi" "EnFlo SW Folder"() -> (w470:path)
                n207 = Build Path(base path=w470, name or relative path=path "ADAM Server/ADAM_scan_table.vi") -> (appended path=w468:path)
                n208 = Open VI Reference(vi path=w468) -> (vi reference=w471:refnum<vi>, error out=w472:errorcluster)  [unwired: 1 in, 4 out]
                n209 = property class="VI"(reference=w471, error in=w472) -> (reference out=w466:refnum<vi>, error out=w465:errorcluster, "Execution:State"=w473:T46)
                n210 = Equal?(x=w473, y=T46."Run top level" ("Execution:State")) -> (x = y?=w467:bool)
                n211 = case shown="False" w467 {
                  tunnel: w466 -> [w478 w495]
                  tunnel: w465 -> [w477 w494]
                  tunnel: [w476 w495] -> w464
                  tunnel: [w475 w494] -> w463
                  frame False {
                    n212 = Two Button Dialog(message="Are you sure that you want to Run the ADAM Scan table on this machine?", 1:"Run" ("F button name (\"Cancel\")"), 2:"Cancel" ("T button name (\"OK\")")) -> (T button?=w479:bool)
                    n213 = case shown="False" w479 {
                      tunnel: w478 -> [w486 w493]
                      tunnel: w477 -> [w485 w492]
                      tunnel: [w484 w493] -> w476
                      tunnel: [w483 w492] -> w475
                      frame False {
                        n214 = property class="VI"(reference=w486, error in=w485, "Front Panel Window:Open"=TRUE) -> (reference out=w490:refnum<vi>, error out=w489:errorcluster)
                        n215 = invoke class="VI" method="Run VI"(reference=w490, error in=w489, "Wait until done"=FALSE, "Auto Dispose Ref"=TRUE) -> (reference out=w484:refnum<vi>, error out=w483:errorcluster)  [unwired: 1 in, 3 out]
                      }
                      frame True {
                      }
                    }
                  }
                  frame True {
                  }
                }
                n216 = event-data() -> ()  [unwired: 1 in, 2 out]
                n217 = Close Reference(reference=w464, error in (no error)=w463) -> ()  [unwired: 1 out]
              }
              event Mouse Down? {
                n218 = event-data() -> ()  [unwired: 5 out]
                n219 = global read "Constants_global.vi" "EnFlo SW Folder"() -> (w498:path)
                n220 = Build Path(base path=w498, name or relative path=path "ADAM Serial/Instrument drivers/Traverses/~subVIs/Read_Write_Trav_Config.vi") -> (appended path=w499:path)
                n221 = Build Path(base path=w498, name or relative path=path "ADAM Serial/Instrument drivers/Traverses/~subVIs/DriveConfigGlobal.vi") -> (appended path=w500:path)
                n222 = flat-sequence {
                  tunnel: w500 -> [w501]
                  tunnel: w499 -> [w503]
                  frame #0 {
                    n223 = call "Open_Close_Front_Panel.ph.vi"("Front Panel Window:Open"=TRUE, "VI path"=w501) -> ()  [unwired: 2 out]
                  }
                  frame #1 {
                    n224 = call "Open_Close_Front_Panel.ph.vi"("Front Panel Window:Open"=TRUE, "VI path"=w503) -> ()  [unwired: 2 out]
                  }
                }
                n225 = event-data() -> ()  [unwired: 1 in, 5 out]
              }
              event Mouse Down? {
                n226 = event-data() -> ()  [unwired: 5 out]
                n227 = global read "Constants_global.vi" "EnFlo SW Folder"() -> (w505:path)
                n228 = Build Path(base path=w505, name or relative path=path "Anemometry/Utilities/Hot_wire_Calculator.vi") -> (appended path=w508:path)
                n229 = call "Open_Close_Front_Panel.ph.vi"("Front Panel Window:Open"=TRUE, "VI path"=w508) -> ()  [unwired: 2 out]
                n230 = event-data() -> ()  [unwired: 1 in, 5 out]
              }
              event "Show Manual Sync": Mouse Down {
                n231 = event-data() -> ()  [unwired: 9 out]
                n232 = global read "Constants_global.vi" "EnFlo SW Folder"() -> (w509:path)
                n233 = Build Path(base path=w509, name or relative path=path "Anemometry/Utilities/EnFlo_Data_Sync_Manual.vi") -> (appended path=w512:path)
                n234 = call "Open_Close_Front_Panel.ph.vi"("Front Panel Window:Open"=TRUE, "VI path"=w512) -> ()  [unwired: 2 out]
              }
              event "Plot_FFID_Calibs.vi": Mouse Down {
                n235 = event-data() -> ()  [unwired: 9 out]
                n236 = global read "Constants_global.vi" "EnFlo SW Folder"() -> (w523:path)
                n237 = Build Path(base path=w523, name or relative path=path "ADAM Client/ADAM client VIs/Plot_FFID_Calibs.vi") -> (appended path=w513:path)
                n238 = Open VI Reference(vi path=w513) -> (vi reference=w516:refnum<vi>, error out=w514:errorcluster)  [unwired: 1 in, 4 out]
                n239 = property class="VI"(reference=w516, error in=w514, "Front Panel Window:Open"=TRUE) -> (reference out=w517:refnum<vi>, error out=w518:errorcluster)
                n240 = invoke class="VI" method="Run VI"(reference=w517, error in=w518, "Wait until done"=FALSE, "Auto Dispose Ref"=TRUE) -> (reference out=w519:refnum<vi>, error out=w520:errorcluster)  [unwired: 1 in, 3 out]
                n241 = Close Reference(reference=w519, error in (no error)=w520) -> ()  [unwired: 1 out]
              }
              event "Beam Check Positions": Mouse Down {
                n242 = event-data() -> ()  [unwired: 9 out]
                n243 = global read "Constants_global.vi" "EnFlo SW Folder"() -> (w535:path)
                n244 = Build Path(base path=w535, name or relative path=path "Anemometry/Anemometry Sub Vis/LDA/Beam_Check_Positions.vi") -> (appended path=w526:path)
                n245 = Open VI Reference(type specifier VI Refnum (for type only)=refnum<vi> refnum, vi path=w526) -> (vi reference=w528:refnum<vi>, error out=w529:errorcluster)  [unwired: 1 in, 3 out]
                n246 = property class="VI Interface Type 4"(reference=w528, error in=w529, "Front Panel Window:Open"=TRUE) -> (reference out=w531:refnum<vi>, error out=w532:errorcluster)
                n247 = call-by-ref "?"(reference=w531, error in=w532, "Mode"=T47."Load From Excel File") -> (reference out=w533:refnum<vi>, error out=w534:errorcluster)  [unwired: 2 in, 1 out]
                n248 = Close Reference(reference=w533, error in (no error)=w534) -> ()  [unwired: 1 out]
              }
              event Mouse Down? {
                n249 = event-data() -> ()  [unwired: 5 out]
                n250 = global read "Constants_global.vi" "EnFlo SW Folder"() -> (w537:path)
                n251 = Build Path(base path=w537, name or relative path=path "Anemometry/Utilities/Hydrosonic_Manual.vi") -> (appended path=w540:path)
                n252 = call "Open_Close_Front_Panel.ph.vi"("Front Panel Window:Open"=TRUE, "VI path"=w540) -> ()  [unwired: 2 out]
                n253 = event-data() -> ()  [unwired: 1 in, 5 out]
              }
              event "Top Level Traverse": Mouse Down {
                n254 = event-data() -> ()  [unwired: 9 out]
                n255 = global read "Constants_global.vi" "EnFlo SW Folder"() -> (w541:path)
                n256 = Build Path(base path=w541, name or relative path=path "Anemometry/Utilities/Top_Level_Move_Traverse.vi") -> (appended path=w544:path)
                n257 = call "Open_Close_Front_Panel.ph.vi"("Front Panel Window:Open"=TRUE, "VI path"=w544) -> ()  [unwired: 2 out]
              }
              event "Post_Pro_Results_Hierarchy": Mouse Down {
                n258 = event-data() -> ()  [unwired: 9 out]
                n259 = global read "Constants_global.vi" "EnFlo SW Folder"() -> (w545:path)
                n260 = Build Path(base path=w545, name or relative path=path "Anemometry/Utilities/Post_Pro_Results_Hierarchy.vi") -> (appended path=w548:path)
                n261 = call "Open_Close_Front_Panel.ph.vi"("Front Panel Window:Open"=TRUE, "VI path"=w548) -> ()  [unwired: 2 out]
              }
              event Mouse Down? {
                n262 = event-data() -> ()  [unwired: 5 out]
                n263 = global read "Constants_global.vi" "EnFlo SW Folder"() -> (w549:path)
                n264 = Build Path(base path=w549, name or relative path=path "ADAM Client/ADAM client VIs/Fast_FID_Valve_Control.vi") -> (appended path=w552:path)
                n265 = call "Open_Close_Front_Panel.ph.vi"("Front Panel Window:Open"=TRUE, "VI path"=w552) -> ()  [unwired: 2 out]
                n266 = event-data() -> ()  [unwired: 1 in, 5 out]
              }
              event Mouse Down? {
                n267 = event-data() -> ()  [unwired: 5 out]
                n268 = global read "Constants_global.vi" "EnFlo SW Folder"() -> (w553:path)
                n269 = Build Path(base path=w553, name or relative path=path "Anemometry/Utilities/Preference_Panel.vi") -> (appended path=w562:path)
                n270 = Open VI Reference(type specifier VI Refnum (for type only)=refnum<vi> refnum, vi path=w562) -> (vi reference=w555:refnum<vi>, error out=w556:errorcluster)  [unwired: 1 in, 3 out]
                n271 = property class="VI Interface Type 1"(reference=w555, error in=w556, "Front Panel Window:Open"=TRUE) -> (reference out=w558:refnum<vi>, error out=w559:errorcluster)
                n272 = call-by-ref "?"(reference=w558, error in=w559, "Mode"=Preference_Mode."Load, Edit then Save") -> (reference out=w560:refnum<vi>, error out=w561:errorcluster)
                n273 = Close Reference(reference=w560, error in (no error)=w561) -> ()  [unwired: 1 out]
                n274 = event-data("Discard?"=TRUE) -> ()  [unwired: 1 in, 4 out]
              }
              event Mouse Down? {
                n275 = event-data() -> ()  [unwired: 5 out]
                n276 = global read "Constants_global.vi" "EnFlo SW Folder"() -> (w569:path)
                n277 = Build Path(base path=w569, name or relative path=path "ADAM Client/Sub VIs/Gas_Setup.vi") -> (appended path=w576:path)
                n278 = Open VI Reference(type specifier VI Refnum (for type only)=refnum<vi> refnum, vi path=w576) -> (vi reference=w572:refnum<vi>, error out=w573:errorcluster)  [unwired: 1 in, 3 out]
                n279 = property class="VI Interface Type 5"(reference=w572, error in=w573, "Front Panel Window:Open"=TRUE) -> (reference out=w577:refnum<vi>, error out=w575:errorcluster)
                n280 = call-by-ref "?"(reference=w577, error in=w575) -> (reference out=w567:refnum<vi>, error out=w566:errorcluster)  [unwired: 9 in]
                n281 = Close Reference(reference=w567, error in (no error)=w566) -> ()  [unwired: 1 out]
                n282 = event-data("Discard?"=TRUE) -> ()  [unwired: 1 in, 4 out]
              }
              event Mouse Down? {
                n283 = event-data() -> ()  [unwired: 5 out]
                n284 = global read "Constants_global.vi" "EnFlo SW Folder"() -> (w581:path)
                n285 = Build Path(base path=w581, name or relative path=path "ADAM Client/Sub VIs/User_Metadata.vi") -> (appended path=w588:path)
                n286 = Open VI Reference(type specifier VI Refnum (for type only)=refnum<vi> refnum, vi path=w588) -> (vi reference=w584:refnum<vi>, error out=w585:errorcluster)  [unwired: 1 in, 3 out]
                n287 = property class="VI Interface Type 5"(reference=w584, error in=w585, "Front Panel Window:Open"=TRUE) -> (reference out=w589:refnum<vi>, error out=w587:errorcluster)
                n288 = call-by-ref "?"(reference=w589, error in=w587) -> (reference out=w579:refnum<vi>, error out=w578:errorcluster)  [unwired: 9 in]
                n289 = Close Reference(reference=w579, error in (no error)=w578) -> ()  [unwired: 1 out]
                n290 = event-data("Discard?"=TRUE) -> ()  [unwired: 1 in, 4 out]
              }
              event Mouse Down? {
                n291 = event-data() -> ()  [unwired: 5 out]
                n292 = global read "Constants_global.vi" "EnFlo SW Folder"() -> (w595:path)
                n293 = Build Path(base path=w595, name or relative path=path "ADAM Client/Sub VIs/EnFlo_Tunnel_Setup.vi") -> (appended path=w598:path)
                n294 = Open VI Reference(type specifier VI Refnum (for type only)=refnum<vi> refnum, vi path=w598) -> (vi reference=w592:refnum<vi>, error out=w591:errorcluster)  [unwired: 1 in, 3 out]
                n295 = call-by-ref "?"(reference=w592, error in=w591) -> (reference out=w594:refnum<vi>, error out=w593:errorcluster)  [unwired: 9 in]
                n296 = Close Reference(reference=w594, error in (no error)=w593) -> ()  [unwired: 1 out]
                n297 = event-data("Discard?"=TRUE) -> ()  [unwired: 1 in, 4 out]
              }
              event Mouse Down? {
                w612 = TRUE  # Show Panel?
                n298 = event-data() -> ()  [unwired: 5 out]
                n299 = global read "Preference_global.vi" "Use New Collision Code"() -> (w602:bool)
                n300 = global read "Constants_global.vi" "EnFlo SW Folder"() -> (w608:path)
                n301 = Select(t=path "Anemometry/Anemometry Sub Vis/Gen Trav/Traverse_Space_for new collision code.vi", s=w602, f=path "Anemometry/Anemometry Sub Vis/Gen Trav/Traverse_Space.vi") -> (s? t:f=w599:path)
                n302 = Build Path(base path=w608, name or relative path=w599) -> (appended path=w610:path)
                n303 = global read "Trav_pos_global.vi" "Default Traverse Setup"() -> (w603:string)
                n304 = Open VI Reference(type specifier VI Refnum (for type only)=refnum<vi> refnum, vi path=w610) -> (vi reference=w611:refnum<vi>, error out=w604:errorcluster)  [unwired: 1 in, 3 out]
                n305 = call-by-ref "?"(reference=w611, error in=w604, "Show Panel?"=w612, "Traverse Setup"=w603) -> (reference out=w606:refnum<vi>, error out=w605:errorcluster)  [unwired: 8 in, 1 out]
                n306 = Close Reference(reference=w606, error in (no error)=w605) -> ()  [unwired: 1 out]
                n307 = event-data("Discard?"=TRUE) -> ()  [unwired: 1 in, 4 out]
              }
              event Mouse Down? {
                n308 = event-data() -> ()  [unwired: 5 out]
                n309 = global read "Constants_global.vi" "EnFlo SW Folder"() -> (w614:path)
                n310 = Build Path(base path=w614, name or relative path=path "Anemometry/Anemometry Sub Vis/Traverse vi's/EnFlo Tunnel specific/Check_EnFlo_Arm.vi") -> (appended path=w616:path)
                n311 = call "Open_Close_Front_Panel.ph.vi"("Front Panel Window:Open"=TRUE, "VI path"=w616) -> ()  [unwired: 2 out]
                n312 = event-data() -> ()  [unwired: 1 in, 2 out]
              }
              event Mouse Down? {
                n313 = event-data() -> ()  [unwired: 5 out]
                n314 = global read "Constants_global.vi" "EnFlo SW Folder"() -> (w624:path)
                n315 = Build Path(base path=w624, name or relative path=path "Anemometry/Anemometry Sub Vis/Gen Trav/3D_Traverse_move.vi") -> (appended path=w621:path)
                n316 = Strip Path(path=w621) -> (name=w620:string)  [unwired: 1 out]
                n317 = Open VI Reference(vi path=w620) -> (vi reference=w622:refnum<vi>, error out=w623:errorcluster)  [unwired: 1 in, 4 out]
                n318 = property class="VI"(reference=w622, error in=w623) -> (reference out=w618:refnum<vi>, error out=w617:errorcluster, "Front Panel Window:Open"=w619:bool)
                n319 = case shown="False" w619 {
                  tunnel: w621 -> [w628 _]
                  tunnel: w618 -> [_ w645]
                  tunnel: w617 -> [_ w644]
                  frame False {
                    w627 = TRUE  # Last Part of Move?
                    n320 = global read "Trav_pos_global.vi" "Work in Tunnel Coordinates?"() -> (w638:T54)
                    n321 = global read "Trav_pos_global.vi" "Default Traverse Setup"() -> (w636:string)
                    n322 = Open VI Reference(type specifier VI Refnum (for type only)=refnum<vi> refnum, vi path=w628) -> (vi reference=w632:refnum<vi>, error out=w633:errorcluster)  [unwired: 1 in, 3 out]
                    n323 = property class="VI Interface Type 6"(reference=w632, error in=w633, "Front Panel Window:Open"=TRUE) -> (reference out=w629:refnum<vi>, error out=w630:errorcluster)
                    n324 = call-by-ref "?"(reference=w629, error in=w630, "Mode"=Trav_mode."Read traverse position", "Extra command String"="", "Work in Tunnel Coordinates"=w638, "Simulate/Run"=User_Specific_mode."Run VI", "Traverse name"=w636, "Last Part of Move?"=w627) -> (reference out=w634:refnum<vi>, error out=w635:errorcluster)  [unwired: 11 in, 3 out]
                    n325 = Close Reference(reference=w634, error in (no error)=w635) -> ()  [unwired: 1 out]
                  }
                  frame True {
                    n326 = property class="VI"(reference=w645, error in=w644, "Front Panel Window:Open"=TRUE) -> (reference out=w643:refnum<vi>, error out=w642:errorcluster)
                    n327 = Close Reference(reference=w643, error in (no error)=w642) -> ()  [unwired: 1 out]
                  }
                }
                n328 = event-data() -> ()  [unwired: 1 in, 5 out]
              }
              event Mouse Down? {
                n329 = event-data() -> ()  [unwired: 5 out]
                n330 = Open VI Reference(vi path="Multi_Run_Prog.vi") -> (vi reference=w651:refnum<vi>, error out=w650:errorcluster)  [unwired: 1 in, 4 out]
                n331 = property class="VI"(reference=w651, error in=w650, "Front Panel Window:Open"=TRUE) -> (reference out=w648:refnum<vi>, error out=w649:errorcluster)
                n332 = Close Reference(reference=w648, error in (no error)=w649) -> (error out=w646:errorcluster)
                n333 = Unbundle By Name(w646) -> ("status"=w653:bool)
                n334 = case shown="True" w653 {
                  frame False {
                  }
                  frame True {
                    n335 = global read "Constants_global.vi" "EnFlo SW Folder"() -> (w661:path)
                    n336 = call "Setup_Filepath.vi"("Setup File Type"=Setup_Filetype."General", "Filename in"="Multi_Run_Filename.txt" ("name or relative path")) -> ("Filename Out"=w654:path)  [unwired: 1 out]
                    n337 = Build Path(base path=w661, name or relative path=path "Anemometry/Multi_Run_Prog.vi") -> (appended path=w660:path)
                    n338 = call "Read_File_Simple.vi"("Filename"=w654) -> ("string"=w659:string)  [unwired: 2 in, 7 out]
                    n339 = String To Path(string=w659) -> (path=w657:path)
                    n340 = call "Does_file_exist_(simple).vi"("Pathname"=w657) -> ("exists?"=w658:bool)
                    n341 = case shown="True" w658 {
                      tunnel: w660 -> [w663 w675]
                      tunnel: w657 -> [_ w673]
                      frame False {
                        n342 = call "Open_Close_Front_Panel.ph.vi"("Front Panel Window:Open"=TRUE, "VI path"=w663) -> ()  [unwired: 2 out]
                      }
                      frame True {
                        n343 = Open VI Reference(type specifier VI Refnum (for type only)=refnum<vi> refnum, vi path=w675) -> (vi reference=w672:refnum<vi>, error out=w671:errorcluster)  [unwired: 1 in, 3 out]
                        n344 = property class="VI Interface Type 7"(reference=w672, error in=w671, "Front Panel Window:Open"=TRUE) -> (reference out=w669:refnum<vi>, error out=w670:errorcluster)
                        n345 = call-by-ref "?"(reference=w669, error in=w670, "Command filename"=w673, "Mode"=T51."Load Command File" ("Setup mode")) -> (reference out=w668:refnum<vi>, error out=w667:errorcluster)  [unwired: 17 in, 1 out]
                        n346 = Close Reference(reference=w668, error in (no error)=w667) -> ()  [unwired: 1 out]
                      }
                    }
                  }
                }
                n347 = event-data() -> ()  [unwired: 1 in, 5 out]
              }
              event Mouse Down? {
                w677 = "Calibration.vi" ("name or relative path")
                n348 = event-data() -> ()  [unwired: 5 out]
                n349 = global read "Constants_global.vi" "EnFlo SW Folder"() -> (w683:path)
                n350 = Open VI Reference(vi path=w677) -> (vi reference=w681:refnum<vi>, error out=w680:errorcluster)  [unwired: 1 in, 4 out]
                n351 = Build Path(base path=w683, name or relative path="Anemometry") -> (appended path=w686:path)
                n352 = property class="VI"(reference=w681, error in=w680, "Front Panel Window:Open"=TRUE) -> (reference out=w678:refnum<vi>, error out=w679:errorcluster)
                n353 = Build Path(base path=w686, name or relative path=w677) -> (appended path=w684:path)
                n354 = Close Reference(reference=w678, error in (no error)=w679) -> (error out=w676:errorcluster)
                n355 = Unbundle By Name(w676) -> ("status"=w685:bool)
                n356 = case shown="True" w685 {
                  tunnel: w684 -> [_ w688]
                  tunnel: w676 -> [_ _]
                  frame False {
                  }
                  frame True {
                    n357 = stacked-sequence {
                      seq-local: [w694 _] -> [_ w701]
                      tunnel: w688 -> [_ w702]
                      frame #0 {
                        n358 = call "Setup_Filepath.vi"("Setup File Type"=Setup_Filetype."Calibration Setups", "Filename in"="Current_Setup.xls") -> ("Filename Out"=w689:path)  [unwired: 1 out]
                        n359 = call "Read_File_Simple.vi"("Filename"=w689) -> ("string"=w698:string)  [unwired: 2 in, 7 out]
                        n360 = Format Into String(format string="Calibration Setup File   %s", w689) -> (resulting string=w692:string)  [unwired: 2 in, 1 out]
                        n361 = call "Get_string_subset.vi"("String Name"=w692, "String to split"=w698, "File Label"="Raw data header") -> ("Output string"=w696:string)  [unwired: 1 in, 1 out]
                        n362 = call "Get_Characters_from_string.vi"("Input string"=w696, "Variable name"="Calib filename") -> ("Value"=w695:string)  [unwired: 1 in, 1 out]
                        n363 = call "String_to_Pathname.vi"("Input String"=w695) -> ("path"=w694:path)
                      }
                      frame #1 {
                        n364 = call "Does_file_exist_(simple).vi"("Pathname"=w701) -> ("exists?"=w700:bool)
                        n365 = case shown="True" w700 {
                          tunnel: w702 -> [w703 w718]
                          tunnel: w701 -> [_ w712]
                          frame False {
                            n366 = call "Open_Close_Front_Panel.ph.vi"("Front Panel Window:Open"=TRUE, "VI path"=w703) -> ()  [unwired: 2 out]
                          }
                          frame True {
                            w710 = TRUE ("Front Panel Window:Open")
                            n367 = Open VI Reference(type specifier VI Refnum (for type only)=refnum<vi> refnum, vi path=w718) -> (vi reference=w716:refnum<vi>, error out=w711:errorcluster)  [unwired: 1 in, 3 out]
                            n368 = property class="VI Interface Type 8"(reference=w716, error in=w711, "Front Panel Window:Open"=w710, "Front Panel Window:Auto Center (Deprecated)"=w710) -> (reference out=w715:refnum<vi>, error out=w714:errorcluster)
                            n369 = call-by-ref "?"(reference=w715, error in=w714, "Mode"=Calib_mode."Setup Front Panel", "Calib file"=w712) -> (reference out=w708:refnum<vi>, error out=w707:errorcluster)  [unwired: 15 in, 3 out]
                            n370 = property class="VI Interface Type 8"(reference=w708, error in=w707, "Front Panel Window:Auto Center (Deprecated)"=FALSE ("Front Panel Window:Auto Center")) -> (reference out=w706:refnum<vi>, error out=w705:errorcluster)
                            n371 = Close Reference(reference=w706, error in (no error)=w705) -> ()  [unwired: 1 out]
                          }
                        }
                      }
                    }
                  }
                }
                n372 = event-data() -> ()  [unwired: 1 in, 5 out]
              }
              event "stop": Mouse Down? {
                n373 = event-data() -> ()  [unwired: 5 out]
                n374 = flat-sequence {
                  frame #0 {
                    n375 = global write "Dynamic_call_global.ph.vi" "EnFlo Hub running?"(FALSE ("EnFlo Hub running?")) -> ()
                  }
                  frame #1 {
                    n376 = Stop(stop? (T)=TRUE) -> ()
                  }
                }
                n377 = event-data() -> ()  [unwired: 1 in, 4 out]
              }
              event "Rig_Control": Value Change {
                n378 = event-data() -> ("OldVal"=w722:cluster{"Ch Name":string, "Boolean":bool}[], "NewVal"=w721:cluster{"Ch Name":string, "Boolean":bool}[])  [unwired: 5 out]
                n379 = for {
                  tunnel: w722 -> [w728] mode=indexing
                  tunnel: w721 -> [w727] mode=indexing
                  n380 = Unbundle By Name(w728) -> ("Ch Name"=w725:string, "Boolean"=w726:bool)
                  n381 = Unbundle By Name(w727) -> ("Boolean"=w724:bool)  [unwired: 1 out]
                  n382 = Not Equal?(x=w726, y=w724) -> (x != y?=w723:bool)
                  n383 = case shown="True" w723 {
                    tunnel: w725 -> [_ w732]
                    tunnel: w724 -> [_ w729]
                    frame False {
                    }
                    frame True {
                      n384 = case shown="False" w729 {
                        tunnel: ["Off" "On"] -> w731
                        tunnel: [0.0 ("f") 1.0 ("t")] -> w730
                        frame False {
                        }
                        frame True {
                        }
                      }
                      n385 = Format Into String(format string="Are you sure you want to turn %s %s?", w732, w731) -> (resulting string=w737:string)  [unwired: 2 in, 1 out]
                      n386 = Format Into String(format string="Make  %s  %s", w732, w731) -> (resulting string=w733:string)  [unwired: 2 in, 1 out]
                      n387 = Two Button Dialog(message=w737, 1:w733, 2:"Cancel" ("T button name (\"OK\")")) -> (T button?=w735:bool)
                      n388 = case shown="False" w735 {
                        tunnel: w732 -> [w744 _]
                        tunnel: w730 -> [w743 _]
                        frame False {
                          n389 = Build Array(w743) -> (w746:dbl[])
                          n390 = Build Array(w744) -> (w745:string[])
                          n391 = call "ASYNC_Adam_client.vi"("Values"=w746, "Channel Names"=w745) -> ()  [unwired: 1 in, 2 out]
                        }
                        frame True {
                        }
                      }
                    }
                  }
                }
              }
            }
          }
        }
        "Numeric" <- w272
      }
      n392 = while {
        shift-left: _ -> [w749]
        shift-right: [w750] -> _
        shift-left: "Initialise" -> [w748]
        shift-right: [w751] -> _
        i -> [w747]
        stop <- TRUE continue-if-true
        n393 = case shown="\"Wait until remote sub vi is opened\"" w748 {
          tunnel: ["End" "Initialise" "Wait for call remote sub vi occurrence" "Check type of VI to launch" w778 "Wait until remote sub vi is opened" "Update opened vis array" "Update opened vis array" "Update opened vis array" "Wait until remote sub vi is opened" "Wait for call remote sub vi occurrence"] -> w751
          tunnel: [w753 w766 w769 errorcluster {"status"=FALSE, "code"=0, "source"=""} ("error out") w774 w789 w819 w836 w851 w891 w911] -> w750
          tunnel: w749 -> [w753 w766 w769 _ w774 w789 _ _ _ w891 w911]
          tunnel: w748 -> [w755 _ _ _ _ _ _ _ _ _ _]
          tunnel: w747 -> [_ _ _ _ _ _ _ _ _ _ _]
          frame "No match", Default {
            n394 = Current VI's Path() -> (path=w756:path)
            n395 = Format Into String(format string="The Case\"%s\" was not Matched\nin VI named\n'%s\"" ("Format String"), w755, w756) -> (resulting string=w759:string)  [unwired: 2 in, 1 out]
            n396 = One Button Dialog(message=w759, button name ("OK")="STOP") -> (true=w757:bool)
            n397 = Stop(stop? (T)=w757) -> ()
          }
          frame "Never run" {
            # "This keeps the Coherent global and DLL reference alive even after all associated vi's are closed and the Hub is stopped (but not closed, that really is game over....)"
            # "These globals are here to make sure they stay in memory\nafter \"Preference Panel\" has finished running"
            n398 = call "Email_With_Log.vi"() -> ()  [unwired: 4 in, 3 out]
            n399 = call "Remember_value.vi"() -> ()  [unwired: 3 in, 1 out]
            n400 = call "Output_Trav_Pos.vi"() -> ()  [unwired: 5 in, 1 out]
            n401 = call "Read_Write_Local_table.vi"() -> ()  [unwired: 3 in, 3 out]
            n402 = call "Overhead_Factor.vi"() -> ()  [unwired: 4 in, 1 out]
            n403 = global read "Trav_pos_global.vi" "Dummy Measurement?"() -> (→"Dummy Measurement":bool)
            n404 = global read "PWAtasksGLOBAL.vi" "Analogue Dev Name"() -> (→"Analogue Dev Name":string)
            n405 = global read "Constants_global.vi" "All_Users"() -> (→"All Users":path)
            n406 = global read "Preference_global.vi" "Rig Setup"() -> (→"Rig Name":string)
            n407 = call "Get DLL version.vi"() -> ()  [unwired: 3 out]
          }
          frame "Initialise" {
            "Iterations" <- 0 ("Iterations")
          }
          frame "Wait for call remote sub vi occurrence" {
            n408 = global read "Dynamic_call_global.ph.vi" "Call Remote Subvi"() -> (w772:refnum<k4>)
            n409 = Wait on Occurrence(2:w772) -> ()  [unwired: 3 out]
          }
          frame "Check type of VI to launch" {
            n410 = global read "Dynamic_call_global.ph.vi" "VI name to launch"() -> (w776:string)
            n411 = Match Pattern(string=w776, regular expression=";") -> (before substring=w773:string, after substring=w775:string)  [unwired: 3 out]
            n412 = case shown="\"Open LDA PWA & An\"" w773 {
              tunnel: ["Open vi" "Open application reference" "Open Analogue input server" w786] -> w778
              tunnel: [w781 w783 w785 w787] -> w777
              tunnel: w776 -> [w781 _ _ _]
              tunnel: w775 -> [_ w783 w785 w787]
              tunnel: w773 -> [_ _ _ w786]
              frame "Other", Default {
              }
              frame "Open Application Reference" {
              }
              frame "Open Analogue Input VI" {
              }
              frame "Open LDA PWA & An" {
              }
            }
            "VI Name" <- w777
          }
          frame "Open application reference" {
            n413 = local read "VI Name"() -> (w790:string)
            n414 = Match Pattern(string=w790, regular expression=";") -> (before substring=w798:string, after substring=w799:string)  [unwired: 3 out]
            n415 = Decimal String To Number(string=w799) -> (number=w800:i32)  [unwired: 3 out]
            n416 = To Unsigned Long Integer(number=w800) -> (unsigned 32bit integer=w797:u32)
            n417 = call "App_Ref_Global.vi"("Mode"=App_Global."Read Global") -> ("Output Array"=w796:T55[])  [unwired: 1 in, 1 out]
            n418 = Open Application Reference(10:w797, 11:w798) -> (0:w791:errorcluster, 3:w795:refnum<vi>)  [unwired: 1 in, 1 out]
            n419 = for {
              tunnel: w796 -> [w802] mode=indexing
              tunnel: w790 -> [w806]
              tunnel: w795 -> [w804]
              tunnel: [w803] -> w794 mode=indexing
              n420 = Unbundle By Name(w802) -> ("Server IP & Port No"=w807:string)
              n421 = Equal?(x=w807, y=w806) -> (x = y?=w805:bool)
              n422 = case shown="False" w805 {
                tunnel: w804 -> [_ w811]
                tunnel: [w808 w810] -> w803
                tunnel: w802 -> [w808 w809]
                frame False {
                }
                frame True {
                  n423 = Bundle By Name(cluster=w809, "Application reference"=w811) -> (w810:T55)
                }
              }
            }
            n424 = global write "Dynamic_call_global.ph.vi" "Error Cluster"(w791) -> ()
            n425 = call "App_Ref_Global.vi"("Input Array"=w794, "Mode"=App_Global."Write to Global") -> ()  [unwired: 2 out]
          }
          frame "Open Analogue input server" {
            n426 = local read "VI Name"() -> (w816:string)
            n427 = call "Get_link_info.vi"("VI Name"=w816) -> ("Path name"=w813:path, "Application reference"=w814:refnum<vi>, "Local Call?"=w815:bool)  [unwired: 1 out]
            n428 = global read "Dynamic_call_global.ph.vi" "Analogue Input"() -> (w818:refnum<vi>)
            n429 = case shown="True" w815 {
              tunnel: w818 -> [w824 w828]
              tunnel: [w820 w827] -> w817
              tunnel: [w823 w826] -> w819
              tunnel: w816 -> [w822 _]
              tunnel: w814 -> [w821 _]
              tunnel: w813 -> [_ w825]
              frame False {
                n430 = Open VI Reference(type specifier VI Refnum (for type only)=w824, application reference (local)=w821, vi path=w822) -> (vi reference=w820:refnum<vi>, error out=w823:errorcluster)  [unwired: 1 in, 2 out]
              }
              frame True {
                n431 = Open VI Reference(type specifier VI Refnum (for type only)=w828, vi path=w825) -> (vi reference=w827:refnum<vi>, error out=w826:errorcluster)  [unwired: 1 in, 3 out]
              }
            }
            n432 = global write "Dynamic_call_global.ph.vi" "Analogue Input"(w817) -> ()
          }
          frame "Open LDA PWA & An" {
            n433 = local read "VI Name"() -> (w833:string)
            n434 = call "Get_link_info.vi"("VI Name"=w833) -> ("Path name"=w830:path, "Application reference"=w831:refnum<vi>, "Local Call?"=w832:bool)  [unwired: 1 out]
            n435 = global read "Dynamic_call_global.ph.vi" "Take LDA PWA & An"() -> (w835:refnum<vi>)
            n436 = case shown="True" w832 {
              tunnel: w835 -> [w841 w845]
              tunnel: [w837 w844] -> w834
              tunnel: [w840 w843] -> w836
              tunnel: w833 -> [w839 _]
              tunnel: w831 -> [w838 _]
              tunnel: w830 -> [_ w842]
              frame False {
                n437 = Open VI Reference(type specifier VI Refnum (for type only)=w841, application reference (local)=w838, vi path=w839) -> (vi reference=w837:refnum<vi>, error out=w840:errorcluster)  [unwired: 1 in, 2 out]
              }
              frame True {
                n438 = Open VI Reference(type specifier VI Refnum (for type only)=w845, vi path=w842) -> (vi reference=w844:refnum<vi>, error out=w843:errorcluster)  [unwired: 1 in, 3 out]
              }
            }
            n439 = global write "Dynamic_call_global.ph.vi" "Take LDA PWA & An"(w834) -> ()
          }
          frame "Open vi" {
            n440 = local read "VI Name"() -> (w850:string)
            n441 = call "Get_link_info.vi"("VI Name"=w850) -> ("Path name"=w849:path, "Application reference"=w848:refnum<vi>, "Local Call?"=w847:bool)  [unwired: 1 out]
            n442 = case shown="\"No Match\", Default" w850 {
              tunnel: [w852 w861 w873] -> w851
              tunnel: w850 -> [w857 w860 w877]
              tunnel: w849 -> [_ _ w874]
              tunnel: w848 -> [_ w859 w876]
              tunnel: w847 -> [_ w858 w875]
              frame "No Match", Default {
                n443 = Format Into String(format string="VI named \"%s\" Not matched" ("Format String"), w857) -> (resulting string=w854:string)  [unwired: 2 in, 1 out]
                n444 = Bundle By Name(cluster=errorcluster {"status"=FALSE, "code"=0, "source"=""} ("error out"), "source"=w854, "status"=TRUE ("Bundle Element")) -> (w852:errorcluster)
              }
              frame "Program_Active_server.vi" {
                n445 = global read "Dynamic_call_global.ph.vi" "Program Active server"() -> (w863:refnum<vi>)
                n446 = case shown="True" w858 {
                  tunnel: w863 -> [w868 w872]
                  tunnel: [w867 w871] -> w862
                  tunnel: [w866 w870] -> w861
                  tunnel: w860 -> [w865 w869]
                  tunnel: w859 -> [w864 _]
                  frame False {
                    n447 = Open VI Reference(type specifier VI Refnum (for type only)=w868, application reference (local)=w864, vi path=w865) -> (vi reference=w867:refnum<vi>, error out=w866:errorcluster)  [unwired: 1 in, 2 out]
                  }
                  frame True {
                    n448 = Open VI Reference(type specifier VI Refnum (for type only)=w872, vi path=w869) -> (vi reference=w871:refnum<vi>, error out=w870:errorcluster)  [unwired: 1 in, 3 out]
                  }
                }
                n449 = global write "Dynamic_call_global.ph.vi" "Program Active server"(w862) -> ()
              }
              frame "GPIB_Server.vi" {
                n450 = global read "Dynamic_call_global.ph.vi" "GPIB_Server.vi"() -> (w879:refnum<vi>)
                n451 = case shown="False" w875 {
                  tunnel: w879 -> [w884 w888]
                  tunnel: [w883 w887] -> w878
                  tunnel: [w882 w886] -> w873
                  tunnel: w877 -> [w880 _]
                  tunnel: w876 -> [w881 _]
                  tunnel: w874 -> [_ w885]
                  frame False {
                    n452 = Open VI Reference(type specifier VI Refnum (for type only)=w884, application reference (local)=w881, vi path=w880) -> (vi reference=w883:refnum<vi>, error out=w882:errorcluster)  [unwired: 1 in, 2 out]
                  }
                  frame True {
                    n453 = Open VI Reference(type specifier VI Refnum (for type only)=w888, vi path=w885) -> (vi reference=w887:refnum<vi>, error out=w886:errorcluster)  [unwired: 1 in, 3 out]
                  }
                }
                n454 = global write "Dynamic_call_global.ph.vi" "GPIB_Server.vi"(w878) -> ()
              }
            }
          }
          frame "Update opened vis array" {
            w893 = TRUE  # Dialog Box
            n455 = local read "VI Name"() -> (w892:string)
            n456 = Unbundle By Name(w891) -> ("status"=w896:bool, "source"=w894:string)
            n457 = case shown="True" w896 {
              tunnel: w891 -> [w898 w907]
              tunnel: [w898 w906] -> w895
              tunnel: w892 -> [w899 w902]
              tunnel: w894 -> [_ w905]
              frame False {
                n458 = global read "Dynamic_call_global.ph.vi" "Opened VIs"() -> (w900:string[])
                n459 = To Upper Case(1:w899) -> (0:w897:string)
                n460 = Build Array (concatenate)(w900, w897) -> (w901:string[])
                n461 = global write "Dynamic_call_global.ph.vi" "Opened VIs"(w901) -> ()
              }
              frame True {
                n462 = Concatenate Strings(w902, " " ("Substring"), w905) -> (w903:string)
                n463 = Bundle By Name(cluster=w907, "source"=w903) -> (w906:errorcluster)
              }
            }
            n464 = call "EnFlo_Error_Handler.vi"("error in (no error)"=w895, "Error Type"="Dynamic Call", "Dialog Box (T)"=w893) -> ()  [unwired: 3 out]
          }
          frame "Wait until remote sub vi is opened" {
            n465 = global read "Dynamic_call_global.ph.vi" "Remote Subvi Opened"() -> (w912:refnum<k4>)
            n466 = local read "Iterations"() -> (w910:i32)
            n467 = Increment(x=w910) -> (x+1=w909:i32)
            n468 = local write "Iterations"(w909) -> ()
            n469 = Set Occurrence(w912) -> ()
          }
        }
      }
      n470 = call "Last_modified_date.vi"("Update Now"=TRUE) -> ("RevisionString"=w42:string)  [unwired: 1 out]
      n471 = global write "Meas_global.vi" "ProgRevisionInfo"(w42) -> ()
      n472 = while {
        i -> [w45]
        stop <- FALSE stop-if-true
        n473 = stacked-sequence {
          tunnel: w45 -> [_ w93 w101]
          frame #0 {
            n474 = global read "Dynamic_call_global.ph.vi" "EnFlo Hub running?"() -> (w49:bool)
            n475 = Equal?(x="Tab Control", y=T40."Adam Table" ("Tab Control")) -> (x = y?=w50:bool)
            n476 = And(x=w50, y=w49) -> (x .and. y?=w48:bool)
            n477 = case shown="True" w48 {
              frame True {
                n478 = local read "List of ADAM channels to view"() -> (w59:string[])
                n479 = local read "List of ADAM control channels"() -> (w62:string[])
                n480 = Build Array (concatenate)(w62, w59) -> (w61:string[])
                n481 = call "Get_Current_Scan_client.vi"("ADAM Ch Names"=w61) -> ("Ch Description Array"=w56:T56[], "Numerical Values"=w60:dbl[])  [unwired: 2 out]
                n482 = Array Size(array=w62) -> (size(s)=w57:i32)
                n483 = Array Subset(array=w56, index=w57) -> (w55:T56[])  [unwired: 1 in]
                n484 = Array Subset(array=w60, index=w57) -> (w54:dbl[])  [unwired: 1 in]
                n485 = for {
                  tunnel: w55 -> [w69] mode=indexing
                  tunnel: [w68] -> w53 mode=indexing
                  tunnel: cluster{"Ch Name":string, "Numeric":dbl} {"Ch Name"="", "Numeric"=0.0} ("Cluster") -> [w67]
                  tunnel: w54 -> [w65] mode=indexing
                  n486 = Unbundle By Name(w69) -> ("Ch Name"=w66:string)
                  n487 = Bundle By Name(cluster=w67, "Ch Name"=w66, "Numeric"=w65) -> (w68:cluster{"Ch Name":string, "Numeric":dbl})
                }
                "Current Values" <- w53
                n488 = for {
                  N: w57 -> [_]
                  tunnel: cluster{"Ch Name":string, "Boolean":bool} {"Ch Name"="", "Boolean"=FALSE} ("Cluster") -> [w76]
                  tunnel: w56 -> [w75] mode=indexing
                  tunnel: w60 -> [w73] mode=indexing
                  tunnel: [w70] -> w63 mode=indexing
                  n489 = Unbundle By Name(w75) -> ("Ch Name"=w74:string)
                  n490 = Greater?(x=w73, y=0.5) -> (0:w71:bool)
                  n491 = Bundle By Name(cluster=w76, "Ch Name"=w74, "Boolean"=w71) -> (w70:cluster{"Ch Name":string, "Boolean":bool})
                }
                n492 = local write "Rig_Control"(w63) -> ()
              }
              frame False {
              }
            }
          }
          frame #1 {
            w91 = 300 ("y")
            n493 = global read "Trav_pos_global.vi" "Sync to server now"() -> (w77:bool)
            n494 = Quotient & Remainder(x=w93, y=86400) -> (x-y*floor(x/y)=w94:i32)  [unwired: 1 out]
            n495 = Quotient & Remainder(x=w93, y=21600) -> (x-y*floor(x/y)=w90:i32)  [unwired: 1 out]
            n496 = Equal?(x=w94, y=w91) -> (x = y?=w88:bool)
            n497 = Equal?(x=w91, y=w90) -> (x = y?=w89:bool)
            n498 = Or(x=w88, y=w89) -> (x .or. y?=w81:bool)
            n499 = Select(t=3 ("Months of History to backup"), s=w88, f=1) -> (s? t:f=w85:i32)
            n500 = global read "Preference_global.vi" "Server Comms"() -> (w83:T41)
            n501 = Equal?(x=w83, y=Server_Comms."Server Link Healthy" ("Server Comms")) -> (x = y?=w82:bool)
            n502 = And(x=w81, y=w82) -> (x .and. y?=w79:bool)
            n503 = Compound Arithmetic op=OR(w77, "Sync to server now", w79) -> (w78:bool)
            n504 = case shown="True" w78 {
              tunnel: w85 -> [_ w96]
              frame False {
              }
              frame True {
                n505 = stacked-sequence {
                  tunnel: w96 -> [w99 _]
                  frame #0 {
                    w97 = TRUE  # Check Updates on Server?
                    w98 = TRUE  # Get all Server Files
                    n506 = call "Backup_Client.vi"("Check Updates on Server?"=w97, "Get all Server Files"=w98, "Months of History to backup"=w99) -> ()  [unwired: 1 out]
                  }
                  frame #1 {
                    w100 = FALSE ("Sync to server now")
                    n507 = local write "Sync to server now"(w100) -> ()
                    n508 = global write "Trav_pos_global.vi" "Sync to server now"(w100) -> ()
                  }
                }
              }
            }
          }
          frame #2 {
            n509 = while {
              shift-right: [w108] -> _
              shift-left: "Start" -> [w110]
              tunnel: w101 -> [w107]
              shift-right: [w106] -> _
              shift-left: _ -> [w105]
              shift-right: [w104] -> _
              shift-left: _ -> [w103]
              stop <- w109 continue-if-true
              n510 = case shown="\"Check LDA enabled\"" w110 {
                selector: w110 -> [w115 _ _ _ _ _ _ _]
                tunnel: [FALSE TRUE TRUE TRUE TRUE FALSE FALSE FALSE] -> w109
                tunnel: ["End" w123 w135 w144 w153 "End" "End" "End"] -> w108
                tunnel: w107 -> [_ _ w133 _ _ _ _ _]
                tunnel: [w112 w122 w129 w140 w158 w211 refnum<vi> refnum ("type specifier VI Refnum (for type only)") w265] -> w106
                tunnel: w105 -> [w112 w122 w129 w140 w158 w190 w246 w265]
                tunnel: [w111 w121 w128 w139 w149 w193 w243 w264] -> w104
                tunnel: w103 -> [w111 w121 w128 w139 w149 _ w243 w264]
                frame "No Match", Default {
                  n511 = Current VI's Path() -> (path=w120:path)
                  n512 = Format Into String(format string="The Case\"%s\" was not Matched\nin VI named\n'%s\"" ("Format String"), w115, w120) -> (resulting string=w117:string)  [unwired: 2 in, 1 out]
                  n513 = One Button Dialog(message=w117, button name ("OK")="STOP") -> (true=w119:bool)
                  n514 = Stop(stop? (T)=w119) -> ()
                }
                frame "Start" {
                  n515 = global read "Dynamic_call_global.ph.vi" "EnFlo Hub running?"() -> (w127:bool)
                  n516 = Select(t="Check loopcount", s=w127, f="End") -> (s? t:f=w123:string)
                }
                frame "Check loopcount" {
                  # "Only update every 10 cycles, which, based on 1000ms delay of outer loop equates to 10s sampling period"
                  # "(i MOD 10 == 0) reformulated to exclude first zero"
                  n517 = Quotient & Remainder(x=w133, y=11) -> (x-y*floor(x/y)=w131:i32)  [unwired: 1 out]
                  n518 = Equal?(x=w131, y=10) -> (x = y?=w130:bool)
                  n519 = Select(t="Check rig setup", s=w130, f="End") -> (s? t:f=w135:string)
                }
                frame "Check rig setup" {
                  n520 = global read "Preference_global.vi" "Rig Setup"() -> (w142:string)
                  n521 = Equal?(x=w142, y="EnFlo_Tunnel") -> (x = y?=w141:bool)
                  n522 = Select(t="Check LDA enabled", s=w141, f="End") -> (s? t:f=w144:string)
                }
                frame "Check LDA enabled" {
                  w155 = 0.5 ("y")
                  w151 = "LDA1:Mains_Power:Enable"
                  n523 = Build Array(w151, "LDA1:System:Enable" ("Desired Ch to Read")) -> (w160:string[])
                  n524 = call "Get_Current_Scan_client.vi"("ADAM Ch Names"=w160) -> ("Numerical Values"=w159:dbl[])  [unwired: 1 in, 2 out]
                  n525 = Index Array(array=w159) -> (element #1=w156:dbl, element #2=w154:dbl)  [unwired: 2 in]
                  n526 = Greater?(x=w156, y=w155) -> (0:w152:bool)
                  n527 = Greater?(x=w154, y=w155) -> (0:w148:bool)
                  n528 = And(x=w152, y=w148) -> (x .and. y?=w150:bool)
                  n529 = case shown="False" w150 {
                    tunnel: [w166 "Run monitor"] -> w153
                    tunnel: w152 -> [w164 _]
                    tunnel: w148 -> [w165 _]
                    tunnel: w151 -> [w162 _]
                    frame False {
                      n530 = Compound Arithmetic op=AND(w165, w164) -> (w163:bool)
                      n531 = case shown="True" w164 {
                        tunnel: ["End" w170] -> w166
                        tunnel: w163 -> [_ w169]
                        tunnel: w162 -> [_ w168]
                        frame False {
                        }
                        frame True {
                          n532 = case shown="False" w169 {
                            tunnel: ["End" "Turn Off Lasers" ("t")] -> w170
                            tunnel: w168 -> [w172 _]
                            frame False {
                              n533 = Build Array(w172) -> (w174:string[])
                              n534 = Build Array(0.0 ("y")) -> (w175:dbl[])
                              n535 = call "ASYNC_Adam_client.vi"("Values"=w175, "Channel Names"=w174) -> ()  [unwired: 1 in, 2 out]
                            }
                            frame True {
                            }
                          }
                        }
                      }
                    }
                    frame True {
                    }
                  }
                }
                frame "Run monitor" {
                  w183 = errorcluster {"status"=FALSE, "code"=0, "source"=""} ("error in (no error)")
                  w193 = string[] ["LDA Laser:Green:Power (mW)", "LDA Laser:Green:LDD current (A)", "LDA Laser:Green:TEC drive (V)", "LDA Laser:Green:TEC temp. (degC)", "LDA Laser:Green:SHG heater (degC)", "LDA Laser:Green:BRF heater (degC)", "LDA Laser:Blue:Power (mW)", "LDA Laser:Blue:LDD current (A)", "LDA Laser:Blue:TEC drive (V)", "LDA Laser:Blue:TEC temp. (degC)", "LDA Laser:Blue:SHG heater (degC)", "LDA Laser:Blue:BRF heater (degC)"]
                  w208 = TRUE  # Don't Bother with check?
                  # "Call by reference to prevent loading of sub-hierarchy for rigs not using LDA. Treating the reference opening in this manner means it only ever has to be done once, and only if all checks are passed."
                  n536 = call-by-ref "Start Asynchronous Call"(reference=w190, error in=w183) -> (error out=w191:errorcluster)  [unwired: 2 in, 5 out]
                  n537 = call-by-ref "Wait On Asynchronous Call"(reference=w190, error in=w183) -> (reference out=w188:refnum<vi>, error out=w192:errorcluster, "GREEN LASER"=w187:T62, "BLUE LASER"=w186:T62, "Initialisation error"=w185:errorcluster, "IO error (first)"=w184:errorcluster)  [unwired: 2 in]
                  n538 = Merge Errors(w191, w192) -> (w189:errorcluster)
                  n539 = case shown="Error" w189 {
                    selector: w189 -> [w223 _]
                    tunnel: [w224 w230] -> w211
                    tunnel: w188 -> [w224 _]
                    tunnel: [w223 w229] -> _
                    tunnel: [w222 w225] -> w210
                    tunnel: [w221 w226] -> w209
                    tunnel: [w220 w228] -> w182
                    tunnel: [w219 w227] -> w181
                    tunnel: w187 -> [w222 _]
                    tunnel: w186 -> [w221 _]
                    tunnel: w185 -> [w220 _]
                    tunnel: w184 -> [w219 _]
                    frame No Error {
                    }
                    frame Error {
                      n540 = Current VI's Path() -> (path=w239:path)
                      n541 = Strip Path(path=w239) -> (stripped path=w240:path)  [unwired: 1 out]
                      n542 = Build Path(base path=w240, name or relative path=path "Anemometry Sub Vis/LDA/Coherent/Lasers monitor ONESHOT.vi") -> (appended path=w237:path)
                      n543 = Open VI Reference(type specifier VI Refnum (for type only)=refnum<vi> refnum, vi path=w237, options=256, error in (no error)=errorcluster {"status"=FALSE, "code"=0, "source"=""}) -> (vi reference=w232:refnum<vi>, error out=w233:errorcluster)  [unwired: 2 in]
                      n544 = call-by-ref "Start Asynchronous Call"(reference=w232, error in=w233) -> (error out=w234:errorcluster)  [unwired: 2 in, 5 out]
                      n545 = call-by-ref "Wait On Asynchronous Call"(reference=w232, error in=w233) -> (reference out=w230:refnum<vi>, error out=w231:errorcluster, "GREEN LASER"=w225:T62, "BLUE LASER"=w226:T62, "Initialisation error"=w228:errorcluster, "IO error (first)"=w227:errorcluster)  [unwired: 2 in]
                      n546 = Merge Errors(w234, w231) -> (w229:errorcluster)
                    }
                  }
                  n547 = Unbundle By Name(w210) -> ("Power (mW)"=w207:sgl, "LDD current (A)"=w206:sgl, "TEC drive (V)"=w205:sgl, "TEC temp. (degC)"=w204:sgl, "SHG heater (degC)"=w203:sgl, "BRF heater (degC)"=w202:sgl)
                  n548 = Unbundle By Name(w209) -> ("Power (mW)"=w201:sgl, "LDD current (A)"=w200:sgl, "TEC drive (V)"=w199:sgl, "TEC temp. (degC)"=w198:sgl, "SHG heater (degC)"=w197:sgl, "BRF heater (degC)"=w196:sgl)
                  n549 = Build Array(w207, w206, w205, w204, w203, w202, w201, w200, w199, w198, w197, w196) -> (w195:sgl[])
                  n550 = Merge Errors(w182, w181) -> (w180:errorcluster)
                  n551 = for {
                    tunnel: w193 -> [w217] mode=indexing
                    tunnel: w195 -> [w216] mode=indexing
                    tunnel: [w214] -> w194 mode=indexing
                    n552 = To Double Precision Float(number=w216) -> (double precision float=w215:dbl)
                    n553 = Bundle By Name(cluster=T42 {"Channel Name"="", "New Value"=0.0} ("Update Scan Value Cluster"), "Channel Name"=w217, "New Value"=w215) -> (w214:T42)
                  }
                  n554 = call "EnFlo_Error_Handler.vi"("error in (no error)"=w180, "Error Type"="LDA1_Monitor", "Dialog Box (T)"=FALSE) -> ()  [unwired: 3 out]
                  n555 = call "Update_Current_Value_client.vi"("Don't Bother with check?"=w208, "Update array in"=w194) -> ()
                }
                frame "Turn Off Lasers" {
                  w245 = TRUE  # Don't Bother with check?
                  w249 = FALSE ("Green Laser on")
                  n556 = for {
                    tunnel: w243 -> [w262] mode=indexing
                    tunnel: [w261] -> w244 mode=indexing
                    n557 = Bundle By Name(cluster=T42 {"Channel Name"="", "New Value"=0.0} ("Update Scan Value Cluster"), "Channel Name"=w262, "New Value"=nan) -> (w261:T42)
                  }
                  n558 = Current VI's Path() -> (path=w253:path)
                  n559 = Strip Path(path=w253) -> (stripped path=w254:path)  [unwired: 1 out]
                  n560 = call "Update_Current_Value_client.vi"("Don't Bother with check?"=w245, "Update array in"=w244) -> ()
                  n561 = Close Reference(reference=w246) -> ()  [unwired: 1 in, 1 out]
                  n562 = Build Path(base path=w254, name or relative path=path "Anemometry Sub Vis/LDA/Coherent/Laser power on,off (simple).vi") -> (appended path=w251:path)
                  n563 = Open VI Reference(type specifier VI Refnum (for type only)=refnum<vi> refnum, vi path=w251, error in (no error)=errorcluster {"status"=FALSE, "code"=0, "source"=""}) -> (vi reference=w257:refnum<vi>, error out=w256:errorcluster)  [unwired: 3 in]
                  n564 = call-by-ref "?"(reference=w257, error in=w256, "Green Laser on"=w249, "Blue Laser on"=w249) -> (reference out=w248:refnum<vi>, error out=w247:errorcluster)  [unwired: 3 out]
                  n565 = Close Reference(reference=w248, error in (no error)=w247) -> ()  [unwired: 1 out]
                }
                frame "End" {
                }
              }
            }
          }
        }
        n566 = Wait (ms)(milliseconds to wait=u32 1000) -> ()  [unwired: 1 out]
      }
    }
  }
